vi "picture_c_labview2014.vi"() -> ()   [LabVIEW 2014]
uses:
  Program Files (x86)/National Instruments/LabVIEW 2017/instr.lib/Lake Shore 336/Lake Shore 336.lvlib
  Program Files (x86)/National Instruments/LabVIEW 2017/instr.lib/Lake Shore 336/Public/Data/Sensor Data (Single Reading).vi
  Program Files (x86)/National Instruments/LabVIEW 2017/instr.lib/Lake Shore 372/Lake Shore 372.lvlib
  <vilib>/Utility/file.llb/Write Delimited Spreadsheet (string).vi
panel:
  out "current time":timestamp format="%<%I:%M:%S %p>T"
  in  "Tab Control":T1(tab)
  out "Reading 372":bool
  out "Reading 336":bool
  out "Arduino OK":bool
  out "Nitrogen tank":waveform(dbl)(graph)={"t0"=timestamp(3512160360.4800687 s since 1904-01-01), "dt"=0.0, "Y"=[0.0]}
  out "Helium tank":waveform(dbl)[](graph)=[{"t0"=timestamp(3512160360.4800687 s since 1904-01-01), "dt"=0.0, "Y"=[0.0]}, {"t0"=timestamp(3512160360.4800687 s since 1904-01-01), "dt"=0.0, "Y"=[0.0]}]
  out "Device (red) and FAA (green)":waveform(dbl)[](graph)=[{"t0"=timestamp(3512160360.6630793 s since 1904-01-01), "dt"=0.0, "Y"=[0.0]}, {"t0"=timestamp(3512160360.6630793 s since 1904-01-01), "dt"=0.0, "Y"=[0.0]}]
  in  "Stop":bool=TRUE
  out "stopping":bool=TRUE
  out "FAA RO600":dbl caption="FAA (K)" min=0.0 max=63200000.0 step=1e-05 format="%_4f"
  out "Sample RuOx":dbl caption="Device (K)" min=0.0 max=63200000.0 step=1e-05 format="%_3f"
  out "Magnet Current (A)":dbl format="%.3f"
  out "4K Diode":dbl format="%_4f"
  out "77K Diode":dbl format="%_4f"
  out "Magnetic Field (kG)":dbl min=-601000.0 max=601000.0 step=0.0001 format="%_3f"
  in  "Auto-Ramp":bool
  in  "ramp start time":timestamp
  out "Ramp Status":string="Shutting down"
  out "Ramp State":u16(ring)=6 items=["Ramp Up", "Soak (hold)", "Ramp Down", "Ramp up to Setpoint", "Closed Loop Feedback", "Ramp down from Setpoint", "Magnet off"]
  out "Magnet Current":waveform(dbl)(graph)={"t0"=timestamp(3512160360.4800687 s since 1904-01-01), "dt"=0.0, "Y"=[0.0]}
  in  "Calculate Autoramp Time":bool
  in  "End of Ramp Temp Control":bool=TRUE
  in  "soak time (minutes)":dbl=30.0
  out "cycle time (min)":dbl format="%#_3g"
  out "Ramp down step size (mA)":dbl=1.0
  in  "setpoint (K)":dbl=0.1
  in  "Manual temp control":bool
  in  "Check Arduino":bool
  in  "ls336":refnum<visa-resource-name>="LS336"
  in  "ls372":refnum<visa-resource-name>="LS372"
  in  "Arduino":refnum<visa-resource-name>="COM4"
  out "Ramp up step size (%)":dbl=0.02
  out "max magnet value(%)":dbl=10.0
  in  "Read LS336":bool=TRUE
  in  "Read LS372":bool=TRUE
  in  "Record Temps":bool=TRUE
  in  "Timeout (ms)":i32=1000
  out "Ramp up step size (mA)":dbl=1.0
  in  "Max current (A)":dbl=9.4
  in  "thermo data path":path=path "C:/Data/temperature_log/pictureC"
  in  "Field constant (kG/A)":dbl=4.589 min=0.001 max=10.0 step=1e-05 format="%.3f"
  out "Ramp down step size (%)":dbl=0.02
  out "ramp up time (min)":dbl=60.0
  out "ramp down time (min)":dbl=60.0
  out "ramp down start time":timestamp
  in  "Ramp up rate (mA/s)":dbl=5.0
  in  "Ramp down rate (mA/s)":dbl=5.0
  in  "Heat Switch":bool
  in  "Ramp Magnet Up":bool
  in  "Ramp Magnet Down":bool
  in  "control channel":string="A"
  out "Arduino Response":string
  in  "Arduino IP":string="10.200.130.3"
  out "Arduino error":errorcluster
  out "counter":dbl
  in  "delay after ramp down (min)":dbl=20.0
  out "counter 2":dbl
  out "ramp finish time":timestamp
  out "Magnet Current (%)":dbl format="%.3f"
  out "Heater Range Set":u16(ring) items=["Off", "31.6 uA", "100 uA", "316 uA", "1.00 mA", "3.16 mA", "10.0 mA", "31.6 mA", "100 mA"]
  out "Heater Range Actual":u16(ring) items=["Off", "31.6 uA", "100 uA", "316 uA", "1.00 mA", "3.16 mA", "10.0 mA", "31.6 mA", "100 mA"]
  out "Magnet Current Multiplier":dbl=1.0
  out "Heater Range OK":bool
  out "actual Setpoint":dbl min=0.0 max=100000000.0 step=1e-06 format="%.5f"
  in  "Channel (1)":u16(ring)=1 items=["1"=1, "2"=2, "3"=3, "4"=4, "5"=5, "6"=6, "7"=7, "8"=8, "9"=9, "10"=10, "11"=11, "12"=12, "13"=13, "14"=14, "15"=15, "16"=16, "A (Control Input)"=17]
  in  "Excitation Range (5: 200 uV / 100 pA)":u16(ring)=5 items=["2.00 uV / 1.00 pA"=1, "6.32 uV / 3.16 pA"=2, "20.0 uV / 10.0 pA"=3, "63.2 uV / 31.6 pA"=4, "200 uV / 100 pA"=5, "632 uV / 316 pA"=6, "2.00 mV / 1.00 nA"=7, "6.32 mV / 3.16 nA"=8, "20.0 mV / 10.0 nA"=9, "63.2 mV / 31.6 nA"=10, "200 mV / 100 nA"=11, "632 mV / 316 nA"=12, "1.00 uA"=13, "3.16 uA"=14, "10.0 uA"=15, "31.6 uA"=16, "100 uA"=17, "316 uA"=18, "1.00 mA"=19, "3.16 mA"=20, "10.0 mA"=21, "31.6 mA"=22]
  in  "Autorange (0: Autorange off)":u16(ring) items=["Autorange off", "Autorange Current", "ROX 102B Autorange"]
  in  "Excitation  (T: On)":bool=TRUE
  in  "Excitation Mode (0: Voltage)":u16(ring) items=["Voltage", "Current"]
  in  "Resistance Range (17: 200 kOhm)":u16(ring)=17 items=["2.00 mOhm"=1, "6.32 mOhm"=2, "20.0 mOhm"=3, "63.2 mOhm"=4, "200 mOhm"=5, "632 mOhm"=6, "2.00 Ohm"=7, "6.32 Ohm"=8, "20.0 Ohm"=9, "63.2 Ohm"=10, "200 Ohm"=11, "632 Ohm"=12, "2.00 kOhm"=13, "6.32 kOhm"=14, "20.0 kOhm"=15, "63.2 kOhm"=16, "200 kOhm"=17, "632 kOhm"=18, "2.00 MOhm"=19, "6.32 MOhm"=20, "20.0 MOhm"=21, "63.2 MOhm"=22]
  in  "Heater ON/OFF":bool
  in  "Warmup Heater Power (W)":dbl min=0.0 max=10.0
  out "Magnet RTD R":dbl caption="Magnet R (Ohms)" format="%.2f"
  out "GGG RO600 R":dbl caption="GGG R (Ohms)" format="%_4f"
  out "GGG RO600":dbl caption="GGG (K)" format="%_4f"
  out "Magnet RTD":dbl caption="Magnet (K)" format="%.2f"
  out "FAA RO600 R":dbl caption="FAA R (Ohms)" min=0.0 max=63200000.0 step=1e-05 format="%_4f"
  out "Sample RuOx R":dbl caption="Device R (Ohms)" min=0.0 max=63200000.0 step=1e-05 format="%_3f"
  out "GGG":waveform(dbl)(graph)={"t0"=timestamp(3512160360.4800687 s since 1904-01-01), "dt"=0.0, "Y"=[0.0]}
  out "magnet":waveform(dbl)(graph)={"t0"=timestamp(3512160360.4800687 s since 1904-01-01), "dt"=0.0, "Y"=[0.0]}
  in  "initialize":bool
  # "PICTURE-C!"
  # "ADR CONTROL"
  # "How often to measure temps?\nDon't change this during ramps."
  # "Ramp Parameters"
  # "\"A\" for Darkness \n\"1\" for MEC"
  # "Manual ADR CONTROL"
  # "OPEN"
  # "CLOSED"
  # "Lakeshore 372"
  # "Thermometers\nUse ~ 20 uV or ~20 nA excitation for FAA and device thermometers. \nHPD recommendations (these are conservative. Scientific instruments used excitations that were 10 to 100 times higher)\nT(K)                            excitation (nA)\n.175 to 4.2                  10\n.1 to .175                    3\n<.1                              0.1\n\nDiodes get 10 uA excitation. \n\n\nIP Addresses: Palomar July 2016 \nArduino at Palomar July 2016      10.200.130.3\nLS372 at Palomar July 2016          10.200.130.1\nLS336 at Palomar July 2016           10.200.130.2\nGateway at Palomar Nov 2016     10.200.1.129\nDARKNESS lab computer (this machine)      10.200.72.36\nsubnet mask                                   255.255.0.0\n\nWhen changing IP addresses for the Lakeshores, open NIMAX and find the lakeshores under Devices and Interfaces>\nNetwork Devices. Select a Lakeshore and go to the TCP/IP tab in the right panel (tabs are at the bottom of the window.).\nChange the IP and click Validate. If the validation works, click Save.  \n\n\nKepco Front Panel\nVoltage Control = OFF\nCurrent Control = OFF\nMode = Voltage\n\nSample Heater Output from LS372 connects to Voltage Programming Input on Kepco. Red terminal on front of Kepco should\nget a voltage <0, Red magnet wire goes to OUT on back of Kepco, Blue wire goes to COM on back of Kepco.\n\n\nArduino\nTo change the ip address of the arduino, open \nC:\\Users\\kids\\Documents\\Arduino\\heatSwitch\\darkness\\heatSwitch_blackLab\\heatSwitch_blackLab.ino\nor\nC:\\Users\\kids\\Documents\\Arduino\\heatSwitch\\darkness\\heatSwitch_blackLab\\heatSwitch_palomar.ino\nand connect the arduino to this computer (darkness.physics.ucsb.edu) and upload the new file.\n\nFor debugging the UDP connection, use \nC:\\Users\\kids\\Documents\\DARKNESS_labview\\arduino_udp_test.vi"
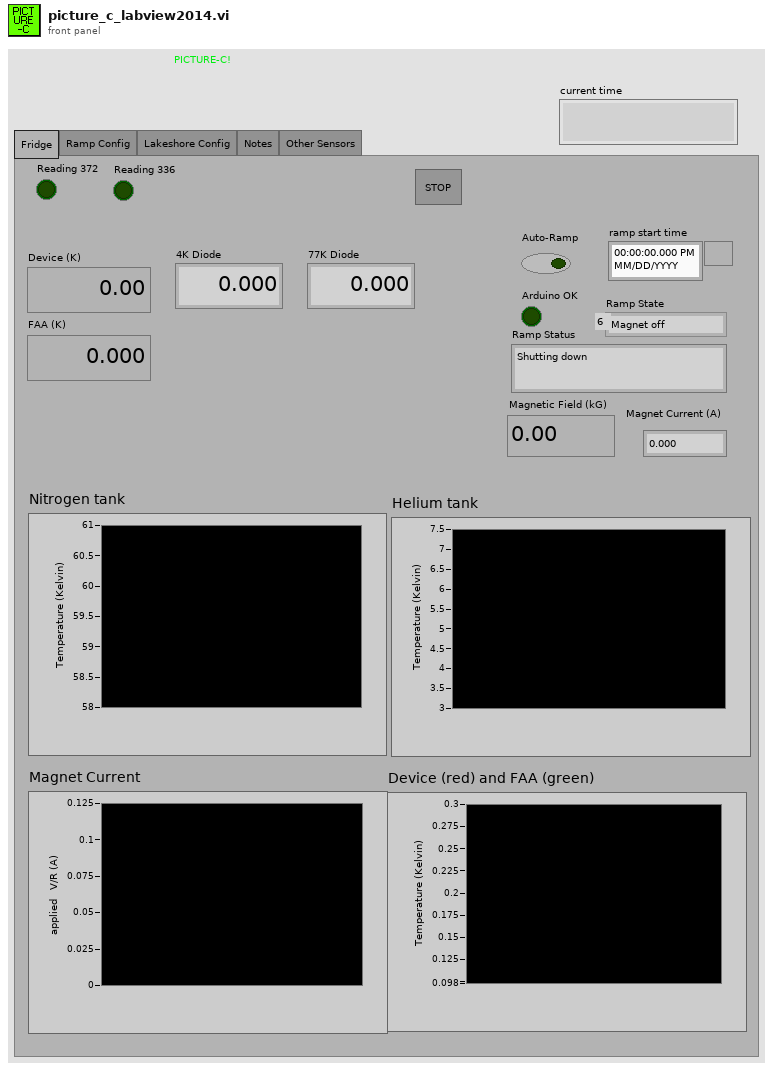
[diagram p1: front panel]
types:
  T1 = enum32{"Fridge", "Ramp Config", "Lakeshore Config", "Notes", "Other Sensors"}
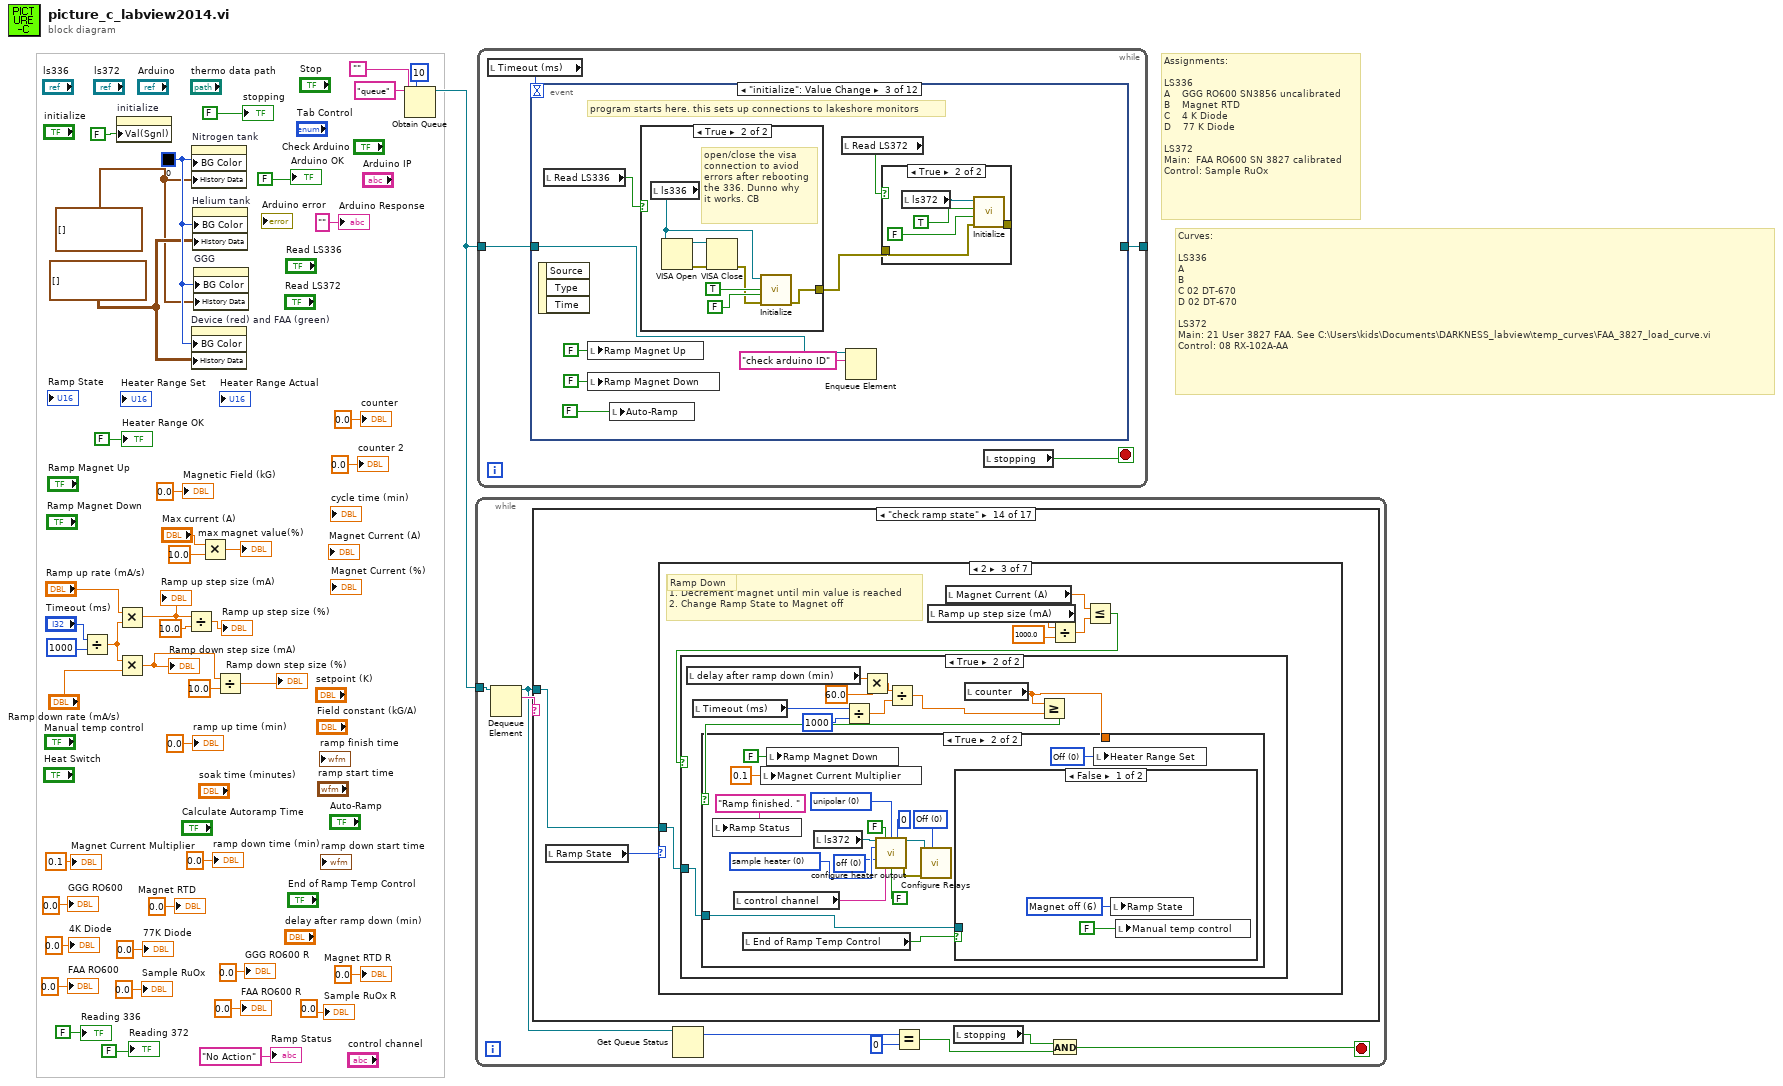
[diagram p0: block diagram]
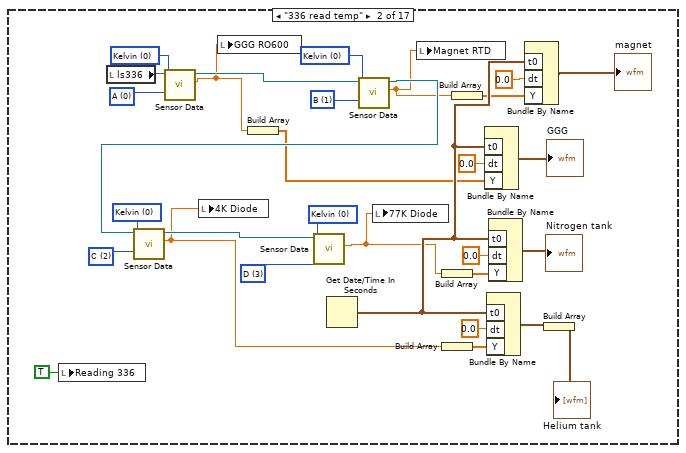
[diagram p3: hidden frame]
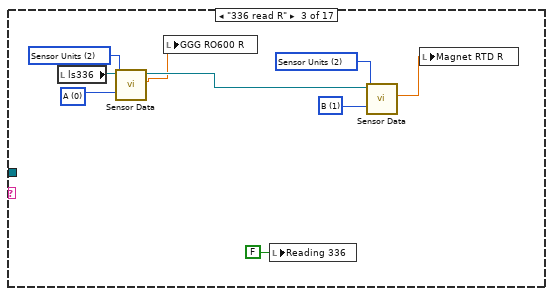
[diagram p4: hidden frame]
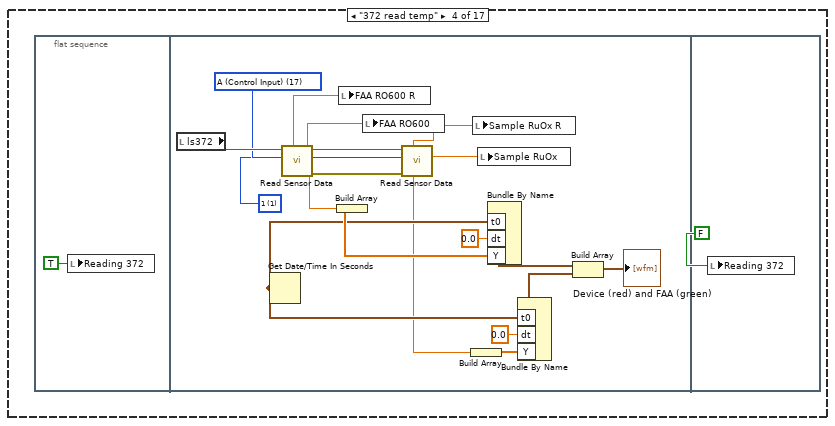
[diagram p5: hidden frame]
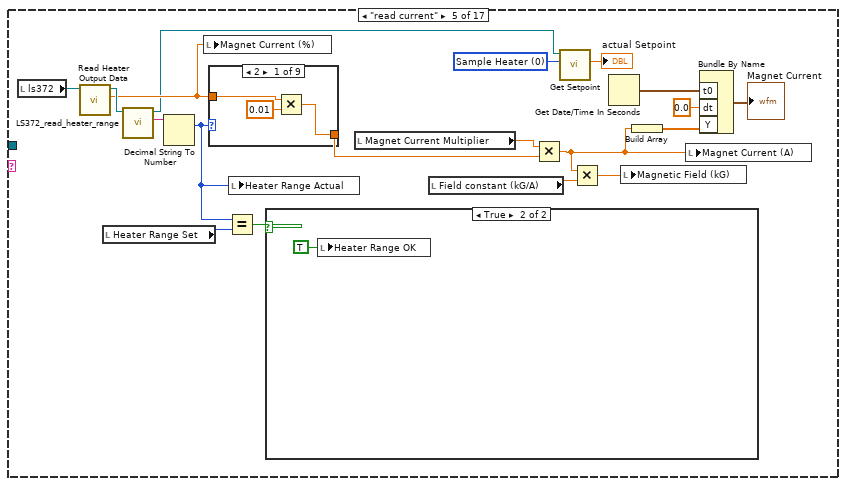
[diagram p6: hidden frame]
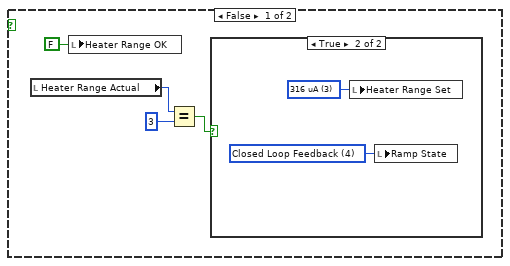
[diagram p7: hidden frame]
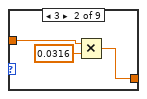
[diagram p9: hidden frame]
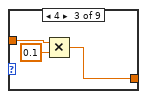
[diagram p10: hidden frame]
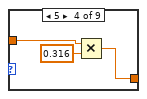
[diagram p11: hidden frame]
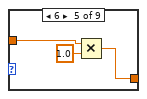
[diagram p12: hidden frame]
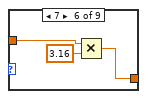
[diagram p13: hidden frame]
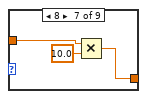
[diagram p14: hidden frame]
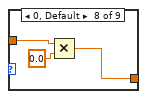
[diagram p15: hidden frame]
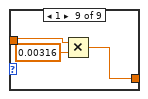
[diagram p16: hidden frame]
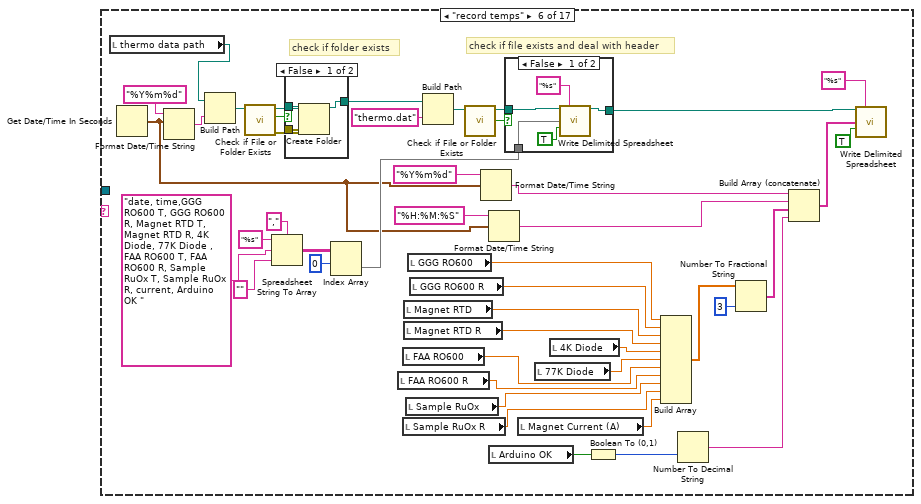
[diagram p17: hidden frame]
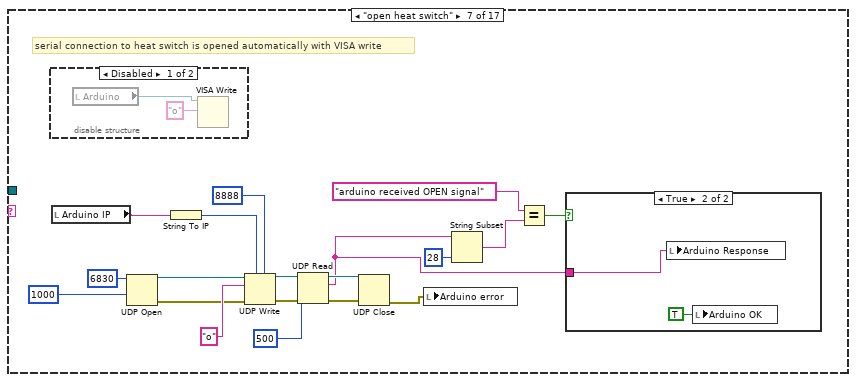
[diagram p20: hidden frame]
diagram:
  w11 = waveform(dbl)[][] [] ("History Data")
  w10 = waveform(dbl)[] [] ("History Data")
  w35 = u32 0
  # "Curves:\n\nLS336\nA\nB\nC 02 DT-670\nD 02 DT-670\n\nLS372\nMain: 21 User 3827 FAA. See C:\\Users\\kids\\Documents\\DARKNESS_labview\\temp_curves\\FAA_3827_load_curve.vi\nControl: 08 RX-102A-AA"
  # "Assignments:\n\nLS336\nA    GGG RO600 SN3856 uncalibrated\nB    Magnet RTD\nC    4 K Diode\nD    77 K Diode\n\nLS372\nMain:  FAA RO600 SN 3827 calibrated\nControl: Sample RuOx"
  n1 = Divide(x="Timeout (ms)", y=1000) -> (x/y=w15:dbl)
  n2 = property on="initialize" class="Bool (strict)"("Val(Sgnl)"=FALSE ("Boolean")) -> ()  [unwired: 2 in, 2 out]
  n3 = Multiply(x="Ramp up rate (mA/s)", y=w15) -> (x*y=w12:dbl)
  "Ramp up step size (mA)" <- w12
  n4 = Multiply(x=w15, y="Ramp down rate (mA/s)") -> (x*y=w13:dbl)
  "Ramp down step size (mA)" <- w13
  n5 = Divide(x=w12, y=10.0) -> (x/y=→"Ramp up step size (%)":dbl)
  n6 = property on="Nitrogen tank" class="WFChart (strict)"("BG Color"=w35, "History Data"=w10) -> ()  [unwired: 2 in, 2 out]
  n7 = property on="Device (red) and FAA (green)" class="WFChart (strict)"("BG Color"=w35, "History Data"=w11) -> ()  [unwired: 2 in, 2 out]
  n8 = property on="Helium tank" class="WFChart (strict)"("BG Color"=w35, "History Data"=w11) -> ()  [unwired: 2 in, 2 out]
  n9 = property on="GGG" class="WFChart (strict)"("BG Color"=w35, "History Data"=w10) -> ()  [unwired: 2 in, 2 out]
  n10 = Multiply(x="Max current (A)", y=10.0) -> (x*y=→"max magnet value(%)":dbl)
  n11 = Divide(x=w13, y=10.0) -> (x/y=→"Ramp down step size (%)":dbl)
  n12 = Obtain Queue(max queue size (-1, unlimited)=10, name (unnamed)="queue", element data type="") -> (queue out=w43:refnum<queue>)  [unwired: 2 in, 2 out]
  n13 = while {
    tunnel: w43 -> [w53]
    stop <- w47 stop-if-true
    n14 = Dequeue Element(queue=w53) -> (queue out=w46:refnum<queue>, element=w52:string)  [unwired: 2 in, 2 out]
    n15 = case shown="\"check ramp state\"" w52 {
      tunnel: w46 -> [_ _ _ _ _ _ _ _ _ _ _ _ _ w477 _ _ _]
      frame "False", Default {
      }
      frame "336 read temp" {
        w74 = u16 0 items=["Kelvin", "Celsius", "Sensor Units"] ("Data Source (0:Kelvin)")
        w75 = u16 3 items=["A", "B", "C", "D"] ("Input (0:A)")
        w77 = u16 0 items=["Kelvin", "Celsius", "Sensor Units"] ("Data Source (0:Kelvin)")
        w78 = u16 2 items=["A", "B", "C", "D"] ("Input (0:A)")
        w80 = u16 0 items=["Kelvin", "Celsius", "Sensor Units"] ("Data Source (0:Kelvin)")
        w81 = u16 1 items=["A", "B", "C", "D"] ("Input (0:A)")
        w82 = u16 0 items=["Kelvin", "Celsius", "Sensor Units"] ("Data Source (0:Kelvin)")
        w83 = u16 0 items=["A", "B", "C", "D"] ("Input (0:A)")
        n16 = local write "Reading 336"(TRUE ("Reading 336")) -> ()
        n17 = local read "ls336"() -> (w84:refnum<visa-resource-name>)
        n18 = call-poly "Sensor Data.vi"("Data Source (0:Kelvin)"=w82, "Input (0:A)"=w83, "VISA resource name"=w84) -> ("Sensor Data"=w62:dbl, "VISA resource name out"=w79:refnum<visa-resource-name>)  [unwired: 6 in, 1 out]
        n19 = local write "GGG RO600"(w62) -> ()
        n20 = Build Array(w62) -> (w63:dbl[])
        n21 = Get Date/Time In Seconds() -> (seconds since 1Jan1904=w67:timestamp)
        n22 = call-poly "Sensor Data.vi"("Data Source (0:Kelvin)"=w80, "Input (0:A)"=w81, "VISA resource name"=w79) -> ("Sensor Data"=w61:dbl, "VISA resource name out"=w76:refnum<visa-resource-name>)  [unwired: 6 in, 1 out]
        n23 = call-poly "Sensor Data.vi"("Data Source (0:Kelvin)"=w77, "Input (0:A)"=w78, "VISA resource name"=w76) -> ("Sensor Data"=w60:dbl, "VISA resource name out"=w73:refnum<visa-resource-name>)  [unwired: 6 in, 1 out]
        n24 = local write "4K Diode"(w60) -> ()
        n25 = call-poly "Sensor Data.vi"("Data Source (0:Kelvin)"=w74, "Input (0:A)"=w75, "VISA resource name"=w73) -> ("Sensor Data"=w59:dbl)  [unwired: 6 in, 2 out]
        n26 = local write "77K Diode"(w59) -> ()
        n27 = local write "Magnet RTD"(w61) -> ()
        n28 = Build Array(w59) -> (w70:dbl[])
        n29 = Build Array(w60) -> (w69:dbl[])
        n30 = Build Array(w61) -> (w64:dbl[])
        n31 = Bundle By Name("t0"=w67, "dt"=0.0, "Y"=w63) -> (→"GGG":waveform(dbl))  [unwired: 1 in]
        n32 = Bundle By Name("t0"=w67, "dt"=0.0, "Y"=w69) -> (w57:waveform(dbl))  [unwired: 1 in]
        n33 = Bundle By Name("t0"=w67, "dt"=0.0, "Y"=w70) -> (→"Nitrogen tank":waveform(dbl))  [unwired: 1 in]
        n34 = Bundle By Name("t0"=w67, "dt"=0.0, "Y"=w64) -> (→"magnet":waveform(dbl))  [unwired: 1 in]
        n35 = Build Array(w57) -> (→"Helium tank":waveform(dbl)[])
      }
      frame "336 read R" {
        w89 = u16 2 items=["Kelvin", "Celsius", "Sensor Units"] ("Data Source (0:Kelvin)")
        w90 = u16 1 items=["A", "B", "C", "D"] ("Input (0:A)")
        w91 = u16 2 items=["Kelvin", "Celsius", "Sensor Units"] ("Data Source (0:Kelvin)")
        w92 = u16 0 items=["A", "B", "C", "D"] ("Input (0:A)")
        n36 = local read "ls336"() -> (w93:refnum<visa-resource-name>)
        n37 = call-poly "Sensor Data.vi"("Data Source (0:Kelvin)"=w91, "Input (0:A)"=w92, "VISA resource name"=w93) -> ("Sensor Data"=w87:dbl, "VISA resource name out"=w88:refnum<visa-resource-name>)  [unwired: 6 in, 1 out]
        n38 = local write "GGG RO600 R"(w87) -> ()
        n39 = local write "Reading 336"(FALSE ("Reading 336")) -> ()
        n40 = call-poly "Sensor Data.vi"("Data Source (0:Kelvin)"=w89, "Input (0:A)"=w90, "VISA resource name"=w88) -> ("Sensor Data"=w86:dbl)  [unwired: 6 in, 2 out]
        n41 = local write "Magnet RTD R"(w86) -> ()
      }
      frame "372 read temp" {
        n42 = flat-sequence {
          frame #0 {
            n43 = local write "Reading 372"(TRUE ("Reading 372")) -> ()
          }
          frame #1 {
            w95 = u16 1 items=["1"=1, "2"=2, "3"=3, "4"=4, "5"=5, "6"=6, "7"=7, "8"=8, "9"=9, "10"=10, "11"=11, "12"=12, "13"=13, "14"=14, "15"=15, "16"=16, "A (Control Input)"=17] ("Channel (1:1)")
            w96 = u16 17 items=["1"=1, "2"=2, "3"=3, "4"=4, "5"=5, "6"=6, "7"=7, "8"=8, "9"=9, "10"=10, "11"=11, "12"=12, "13"=13, "14"=14, "15"=15, "16"=16, "A (Control Input)"=17] ("Channel (1:1)")
            n44 = local read "ls372"() -> (w111:refnum<visa-resource-name>)
            n45 = Get Date/Time In Seconds() -> (seconds since 1Jan1904=w101:timestamp)
            n46 = call "Read Sensor Data.vi"("Channel (1:1)"=w95, "VISA resource name"=w111) -> ("error out"=w109:errorcluster, "Kelvin Reading"=w100:dbl, "Resistance Reading"=w97:dbl, "VISA resource name out"=w110:refnum<visa-resource-name>)  [unwired: 4 in, 2 out]
            n47 = Build Array(w100) -> (w106:dbl[])
            n48 = local write "FAA RO600 R"(w97) -> ()
            n49 = local write "FAA RO600"(w100) -> ()
            n50 = call "Read Sensor Data.vi"("error in (no error)"=w109, "Channel (1:1)"=w96, "VISA resource name"=w110) -> ("Kelvin Reading"=w99:dbl, "Resistance Reading"=w98:dbl)  [unwired: 3 in, 4 out]
            n51 = Build Array(w99) -> (w103:dbl[])
            n52 = local write "Sample RuOx R"(w98) -> ()
            n53 = local write "Sample RuOx"(w99) -> ()
            n54 = Bundle By Name("t0"=w101, "dt"=0.0, "Y"=w106) -> (w107:waveform(dbl))  [unwired: 1 in]
            n55 = Bundle By Name("t0"=w101, "dt"=0.0, "Y"=w103) -> (w102:waveform(dbl))  [unwired: 1 in]
            n56 = Build Array(w107, w102) -> (→"Device (red) and FAA (green)":waveform(dbl)[])
          }
          frame #2 {
            n57 = local write "Reading 372"(FALSE ("Reading 372")) -> ()
          }
        }
      }
      frame "read current" {
        w119 = u16 0 items=["Sample Heater", "Warm-up Heater (Output 1)"] ("Output (0:Sample Heater)")
        n58 = local read "ls372"() -> (w129:refnum<visa-resource-name>)
        n59 = call "Read Heater Output Data.vi"("VISA resource name"=w129) -> ("Heater Output"=w123:dbl, "VISA resource name out"=w128:refnum<visa-resource-name>)  [unwired: 8 in, 1 out]
        n60 = local read "Heater Range Set"() -> (w125:u16)
        n61 = call "LS372_read_heater_range.vi"("VISA resource name"=w128) -> ("heater range"=w127:string, "VISA resource name out"=w118:refnum<visa-resource-name>)  [unwired: 9 in]
        n62 = Decimal String To Number(string=w127) -> (number=w126:i32)  [unwired: 2 in, 1 out]
        n63 = local write "Magnet Current (%)"(w123) -> ()
        n64 = case shown="2" w126 {
          tunnel: [w139 w142 w145 w148 w151 w154 w157 w160 w164] -> w121
          tunnel: w123 -> [w140 w143 w146 w149 w152 w155 w158 w161 w163]
          frame 2 {
            n65 = Multiply(x=w140, y=0.01) -> (x*y=w139:dbl)
          }
          frame 3 {
            n66 = Multiply(x=w143, y=0.0316) -> (x*y=w142:dbl)
          }
          frame 4 {
            n67 = Multiply(x=w146, y=0.1) -> (x*y=w145:dbl)
          }
          frame 5 {
            n68 = Multiply(x=w149, y=0.316) -> (x*y=w148:dbl)
          }
          frame 6 {
            n69 = Multiply(x=w152, y=1.0) -> (x*y=w151:dbl)
          }
          frame 7 {
            n70 = Multiply(x=w155, y=3.16) -> (x*y=w154:dbl)
          }
          frame 8 {
            n71 = Multiply(x=w158, y=10.0) -> (x*y=w157:dbl)
          }
          frame 0, Default {
            n72 = Multiply(x=w161, y=0.0) -> (x*y=w160:dbl)
          }
          frame 1 {
            n73 = Multiply(x=w163, y=0.00316) -> (x*y=w164:dbl)
          }
        }
        n74 = Equal?(x=w126, y=w125) -> (x = y?=w124:bool)
        n75 = local write "Heater Range Actual"(w126) -> ()
        n76 = case shown="True" w124 {
          frame False {
            n77 = local read "Heater Range Actual"() -> (w132:u16)
            n78 = local write "Heater Range OK"(FALSE ("Heater Range OK")) -> ()
            n79 = Equal?(x=w132, y=u16 3) -> (x = y?=w134:bool)
            n80 = case shown="True" w134 {
              frame False {
              }
              frame True {
                w136 = u16 3 items=["Off", "31.6 uA", "100 uA", "316 uA", "1.00 mA", "3.16 mA", "10.0 mA", "31.6 mA", "100 mA"] ("Heater Range Set")
                w137 = u16 4 items=["Ramp Up", "Soak (hold)", "Ramp Down", "Ramp up to Setpoint", "Closed Loop Feedback", "Ramp down from Setpoint", "Magnet off"] ("Ramp State")
                n81 = local write "Heater Range Set"(w136) -> ()
                n82 = local write "Ramp State"(w137) -> ()
              }
            }
          }
          frame True {
            n83 = local write "Heater Range OK"(TRUE ("Heater Range OK")) -> ()
          }
        }
        n84 = local read "Magnet Current Multiplier"() -> (w122:dbl)
        n85 = local read "Field constant (kG/A)"() -> (w131:dbl)
        n86 = Multiply(x=w122, y=w121) -> (x*y=w113:dbl)
        n87 = call "Get Setpoint.vi"("Output (0:Sample Heater)"=w119, "VISA resource name"=w118) -> ("Setpoint (0.00000E+0)"=→"actual Setpoint":dbl)  [unwired: 7 in, 2 out]
        n88 = Multiply(x=w113, y=w131) -> (x*y=w130:dbl)
        n89 = Get Date/Time In Seconds() -> (seconds since 1Jan1904=w117:timestamp)
        n90 = local write "Magnetic Field (kG)"(w130) -> ()
        n91 = Build Array(w113) -> (w116:dbl[])
        n92 = local write "Magnet Current (A)"(w113) -> ()
        n93 = Bundle By Name("t0"=w117, "dt"=0.0, "Y"=w116) -> (→"Magnet Current":waveform(dbl))  [unwired: 1 in]
      }
      frame "record temps" {
        # "check if file exists and deal with header"
        # "check if folder exists"
        n94 = local read "thermo data path"() -> (w186:path)
        n95 = Get Date/Time In Seconds() -> (seconds since 1Jan1904=w176:timestamp)
        n96 = Format Date/Time String(time format string (%c)="%Y%m%d", seconds (now)=w176) -> (date/time string=w198:string)  [unwired: 1 in]
        n97 = Build Path(base path=w186, name or relative path=w198) -> (appended path=w201:path)
        n98 = call <vilib>:"Check if File or Folder Exists.vi"("path"=w201) -> ("error out"=w204:errorcluster, "file or folder exists?"=w203:bool, "dup path"=w202:path)  [unwired: 8 in]
        n99 = Spreadsheet String To Array(delimiter (Tab)=",", format string="%s", spreadsheet string="date, time,GGG RO600 T, GGG RO600 R, Magnet RTD T, Magnet RTD R, 4K Diode, 77K Diode , FAA RO600 T, FAA RO600 R, Sample RuOx T, Sample RuOx R, current, Arduino OK ", array type (2D Dbl)="") -> (array=w184:string[][])
        n100 = case shown="False" w203 {
          tunnel: w202 -> [w219 w220]
          tunnel: w204 -> [w218 _]
          tunnel: [w217 w220] -> w205
          frame False {
            n101 = Create Folder(path (use dialog)=w219, error in=w218) -> (created path=w217:path)  [unwired: 1 in, 2 out]
          }
          frame True {
          }
        }
        n102 = Index Array(array=w184, index (row)=0) -> (element=w178:string[])  [unwired: 1 in]
        n103 = local read "FAA RO600 R"() -> (w189:dbl)
        n104 = local read "FAA RO600"() -> (w190:dbl)
        n105 = local read "Sample RuOx R"() -> (w187:dbl)
        n106 = local read "Magnet RTD"() -> (w194:dbl)
        n107 = local read "Magnet RTD R"() -> (w193:dbl)
        n108 = local read "Sample RuOx"() -> (w188:dbl)
        n109 = local read "GGG RO600"() -> (w210:dbl)
        n110 = local read "GGG RO600 R"() -> (w195:dbl)
        n111 = Build Path(base path=w205, name or relative path="thermo.dat") -> (appended path=w206:path)
        n112 = call <vilib>:"Check if File or Folder Exists.vi"("path"=w206) -> ("file or folder exists?"=w207:bool, "dup path"=w208:path)  [unwired: 8 in, 1 out]
        n113 = Format Date/Time String(time format string (%c)="%Y%m%d", seconds (now)=w176) -> (date/time string=w174:string)  [unwired: 1 in]
        n114 = Format Date/Time String(time format string (%c)="%H:%M:%S", seconds (now)=w176) -> (date/time string=w173:string)  [unwired: 1 in]
        n115 = local read "Arduino OK"() -> (w185:bool)
        n116 = case shown="False" w207 {
          tunnel: [w212 w216] -> w209
          tunnel: w208 -> [w213 w216]
          tunnel: w178 -> [w211 _]
          frame False {
            n117 = call-poly <vilib>:"Write Delimited Spreadsheet.vi"("file path (dialog if empty)"=w213, "format (%s)"="%s" ("format (%.3f)"), "1D data"=w211, "append to file? (new file:F)"=TRUE) -> ("new file path (Not A Path if cancelled)"=w212:path)  [unwired: 10 in, 1 out]
          }
          frame True {
          }
        }
        n118 = local read "Magnet Current (A)"() -> (w196:dbl)
        n119 = local read "77K Diode"() -> (w191:dbl)
        n120 = local read "4K Diode"() -> (w192:dbl)
        n121 = Boolean To (0,1)(Boolean=w185) -> (0, 1=w167:i16)
        n122 = Build Array(w210, w195, w194, w193, w192, w191, w190, w189, w188, w187, w196) -> (w171:dbl[])
        n123 = Number To Decimal String(number=w167) -> (decimal integer string=w166:string)  [unwired: 1 in]
        n124 = Number To Fractional String(number=w171, precision (6)=i16 3) -> (F-format string=w170:string[])  [unwired: 2 in]
        n125 = Build Array (concatenate)(w174, w173, w170, w166) -> (w169:string[])
        n126 = call-poly <vilib>:"Write Delimited Spreadsheet.vi"("file path (dialog if empty)"=w209, "format (%s)"="%s" ("format (%.3f)"), "1D data"=w169, "append to file? (new file:F)"=TRUE) -> ()  [unwired: 10 in, 2 out]
      }
      frame "open heat switch" {
        # "serial connection to heat switch is opened automatically with VISA write"
        n127 = disable-structure shown="Disabled" {
          frame Disabled {
            n128 = local read "Arduino"() -> (w244:refnum<visa-resource-name>)
            n129 = VISA Write(VISA resource name=w244, write buffer="o") -> ()  [unwired: 1 in, 3 out]
          }
          frame Enabled {
          }
        }
        n130 = local read "Arduino IP"() -> (w228:string)
        n131 = UDP Open(9:1000 ("timeout ms (25000)"), 11:u16 6830 ("port")) -> (port=w230:refnum<k16>, 0:w231:errorcluster)  [unwired: 3 in, 1 out]
        n132 = String To IP(1:w228) -> (0:w232:u32)
        n133 = UDP Write(address=w232, port or service name=u16 8888, connection ID=w230, data in="o", 8:w231) -> (error out=w236:errorcluster, 3:w235:refnum<k16>)  [unwired: 1 in]
        n134 = UDP Read(connection ID=w235, timeout ms (25000)=500, 8:w236) -> (data out=w221:string, error out=w239:errorcluster, 3:w238:refnum<k16>)  [unwired: 1 in, 2 out]
        n135 = UDP Close(connection ID=w238, 8:w239) -> (error out=w227:errorcluster)  [unwired: 1 out]
        n136 = local write "Arduino error"(w227) -> ()
        n137 = String Subset(string=w221, length (rest)=28 ("length (rest)")) -> (substring=w222:string)  [unwired: 1 in]
        n138 = Equal?(x="arduino received OPEN signal", y=w222) -> (x = y?=w225:bool)
        n139 = case shown="True" w225 {
          tunnel: w221 -> [_ w242]
          frame False {
            n140 = local write "Arduino Response"("did not respond" ("Arduino Response")) -> ()
            n141 = local write "Arduino OK"(FALSE ("Arduino OK")) -> ()
          }
          frame True {
            n142 = local write "Arduino Response"(w242) -> ()
            n143 = local write "Arduino OK"(TRUE ("Arduino OK")) -> ()
          }
        }
      }
      frame "close heat switch" {
        n144 = local read "Ramp State"() -> (w246:u16)
        n145 = local read "Arduino IP"() -> (w254:string)
        n146 = UDP Open(9:1000 ("timeout ms (25000)"), 11:u16 6830 ("port")) -> (port=w256:refnum<k16>, 0:w257:errorcluster)  [unwired: 3 in, 1 out]
        n147 = case shown="4" w246 {
          frame 0, Default {
          }
          frame 4 {
            w276 = u16 0 items=["unipolar", "bipolar"] ("polarity")
            w277 = u16 0 items=["Off", "31.6 uA", "100 uA", "316 uA", "1.00 mA", "3.16 mA", "10.0 mA", "31.6 mA", "100 mA"] ("Heater Range Set")
            w278 = u16 6 items=["Ramp Up", "Soak (hold)", "Ramp Down", "Ramp up to Setpoint", "Closed Loop Feedback", "Ramp down from Setpoint", "Magnet off"] ("Ramp State")
            w280 = u16 0 items=["sample heater", "output 1 (warm-up heater) ", "output 2 (analog/still)"] ("Output (0: sample heater)")
            w279 = u16 0 items=["off", "monitor out", "open loop (manual)", "zone", "still", "closed loop (PID)", "warmup"] ("mode")
            n148 = local read "ls372"() -> (w270:refnum<visa-resource-name>)
            n149 = Get Date/Time String() -> (time string=w268:string)  [unwired: 3 in, 1 out]
            n150 = Concatenate Strings("heat switch closed at " ("Ramp Status"), w268) -> (w267:string)
            n151 = call "Configure Setpoint.vi"("Setpoint (0.00000E+0)"=0.01, "VISA resource name"=w270) -> ("VISA resource name out"=w269:refnum<visa-resource-name>)  [unwired: 8 in, 1 out]
            n152 = local read "control channel"() -> (w272:string)
            n153 = local write "Ramp Status"(w267) -> ()
            n154 = call "configure heater output.vi"("VISA resource name"=w269, "power up enable"=FALSE, "polarity"=w276, "delay"=0, "Output (0: sample heater)"=w280, "mode"=w279, "input/channel"=w272, "filter"=FALSE) -> ()  [unwired: 6 in, 2 out]
            n155 = local write "Heater Range Set"(w277) -> ()
            n156 = local write "Ramp State"(w278) -> ()
          }
        }
        n157 = String To IP(1:w254) -> (0:w258:u32)
        n158 = UDP Write(address=w258, port or service name=u16 8888, connection ID=w256, data in="c", 8:w257) -> (error out=w262:errorcluster, 3:w261:refnum<k16>)  [unwired: 1 in]
        n159 = UDP Read(connection ID=w261, timeout ms (25000)=500, 8:w262) -> (data out=w247:string, error out=w265:errorcluster, 3:w264:refnum<k16>)  [unwired: 1 in, 2 out]
        n160 = UDP Close(connection ID=w264, 8:w265) -> (error out=w253:errorcluster)  [unwired: 1 out]
        n161 = String Subset(string=w247, length (rest)=29 ("length (rest)")) -> (substring=w248:string)  [unwired: 1 in]
        n162 = local write "Arduino error"(w253) -> ()
        n163 = Equal?(x="arduino received CLOSE signal", y=w248) -> (x = y?=w251:bool)
        n164 = case shown="True" w251 {
          tunnel: w247 -> [_ w283]
          frame False {
            n165 = local write "Arduino Response"("did not respond" ("Arduino Response")) -> ()
            n166 = local write "Arduino OK"(FALSE ("Arduino OK")) -> ()
          }
          frame True {
            n167 = local write "Arduino Response"(w283) -> ()
            n168 = local write "Arduino OK"(TRUE ("Arduino OK")) -> ()
          }
        }
      }
      frame "check arduino ID" {
        # "string received from arduino probably has \\r\\n or \nor something at end, so only look at first 25 \ncharacters"
        n169 = local read "Arduino IP"() -> (w293:string)
        n170 = String To IP(1:w293) -> (0:w297:u32)
        n171 = UDP Open(9:1000 ("timeout ms (25000)"), 11:u16 8888 ("port")) -> (port=w295:refnum<k16>, 0:w296:errorcluster)  [unwired: 3 in, 1 out]
        n172 = UDP Write(address=w297, port or service name=u16 8888, connection ID=w295, data in="I", 8:w296) -> (error out=w300:errorcluster, 3:w299:refnum<k16>)  [unwired: 1 in]
        n173 = UDP Read(connection ID=w299, timeout ms (25000)=500, 8:w300) -> (data out=w289:string, error out=w303:errorcluster, 3:w302:refnum<k16>)  [unwired: 1 in, 2 out]
        n174 = UDP Close(connection ID=w302, 8:w303) -> (error out=w286:errorcluster)  [unwired: 1 out]
        n175 = String Subset(string=w289, length (rest)=25 ("length (rest)")) -> (substring=w287:string)  [unwired: 1 in]
        n176 = local write "Arduino error"(w286) -> ()
        n177 = Equal?(x="arduino says hello world!", y=w287) -> (x = y?=w290:bool)
        n178 = case shown="False" w290 {
          tunnel: w289 -> [_ w307]
          frame False {
            n179 = local write "Arduino Response"("did not respond" ("Arduino Response")) -> ()
            n180 = local write "Arduino OK"(FALSE ("Arduino OK")) -> ()
          }
          frame True {
            n181 = local write "Arduino Response"(w307) -> ()
            n182 = local write "Arduino OK"(TRUE ("Arduino OK")) -> ()
          }
        }
      }
      frame "initialize ramp up" {
        w311 = u16 1 items=["Off", "On", "Alarms", "Sample Heater Zone", "Warmup Heater Zone"] ("Relay Mode (0: Off)")
        w323 = u16 0 items=["sample heater", "output 1 (warm-up heater) ", "output 2 (analog/still)"] ("Output (0: sample heater)")
        w319 = u16 0 items=["unipolar", "bipolar"] ("polarity")
        w317 = u16 2 items=["off", "monitor out", "open loop (manual)", "zone", "still", "closed loop (PID)", "warmup"] ("mode")
        w316 = u16 0 items=["sample heater", "output 1 (warm-up heater) ", "output 2 (analog/still)"] ("Output (0: sample heater)")
        # "Start the magnet ramping up. Check whether starting ramp from 0 (what if labview crashes while\nmagnet is ramping up?)"
        n183 = local read "Ramp up step size (mA)"() -> (w329:dbl)
        n184 = local read "ls372"() -> (w328:refnum<visa-resource-name>)
        n185 = call "Read Heater Output Data.vi"("VISA resource name"=w328) -> ("error out"=w315:errorcluster, "Heater Output"=w332:dbl, "VISA resource name out"=w314:refnum<visa-resource-name>)  [unwired: 8 in]
        n186 = Divide(x=w329, y=100.0) -> (x/y=w327:dbl)
        n187 = local write "Magnet Current Multiplier"(25.66 ("Magnet Current Multiplier")) -> ()
        n188 = Less Or Equal?(x=w332, y=w327) -> (x <= y?=w330:bool)
        n189 = Select(t=0.0, s=w330, f=w332) -> (s? t:f=w313:dbl)
        n190 = local read "Heater Range Set"() -> (w312:u16)
        n191 = call "configure heater output.vi"("VISA resource name"=w314, "power up enable"=FALSE, "polarity"=w319, "delay"=0, "Output (0: sample heater)"=w316, "mode"=w317, "error in (no error)"=w315, "input/channel"="A", "filter"=FALSE) -> ("VISA resource name out"=w324:refnum<visa-resource-name>, "error out"=w325:errorcluster)  [unwired: 5 in]
        n192 = call "Configure Control Parameters.vi"("VISA resource name"=w324, "Output (0: sample heater)"=w323, "Manual Output (0.000%)"=w313, "Heater Range (0: Off)"=w312, "error in (no error)"=w325) -> ("VISA resource name out"=w310:refnum<visa-resource-name>, "error out"=w309:errorcluster)  [unwired: 9 in]
        n193 = call "Configure Relays.vi"("Relay Mode (0: Off)"=w311, "error in (no error)"=w309, "VISA resource name"=w310) -> ()  [unwired: 7 in, 2 out]
      }
      frame "set up autoramp times" {
        n194 = local read "current time"() -> (w334:timestamp)
        n195 = local read "ramp start time"() -> (w333:timestamp)
        n196 = Greater?(x=w334, y=w333) -> (0:w335:bool)
        n197 = case shown="True" w335 {
          frame True {
            n198 = Get Date/Time In Seconds() -> (seconds since 1Jan1904=w369:timestamp)
            n199 = local read "Ramp down rate (mA/s)"() -> (w348:dbl)
            n200 = local read "Max current (A)"() -> (w355:dbl)
            n201 = local read "Ramp up rate (mA/s)"() -> (w352:dbl)
            n202 = local read "Timeout (ms)"() -> (w367:i32)
            n203 = local read "Timeout (ms)"() -> (w362:i32)
            n204 = local read "Max current (A)"() -> (w349:dbl)
            n205 = Add(x=w369, y=10.0) -> (x+y=w342:timestamp)
            n206 = local write "ramp start time"(w342) -> ()
            n207 = Divide(x=w367, y=1000) -> (x/y=w365:dbl)
            n208 = Divide(x=w362, y=1000) -> (x/y=w364:dbl)
            n209 = Multiply(x=w355, y=1000.0) -> (x*y=w353:dbl)
            n210 = Multiply(x=w349, y=1000.0) -> (x*y=w351:dbl)
            n211 = Divide(x=w353, y=w352) -> (x/y=w340:dbl)
            n212 = Multiply(x=w352, y=w365) -> (x*y=w357:dbl)
            n213 = Multiply(x=w348, y=w364) -> (x*y=w356:dbl)
            n214 = Divide(x=w351, y=w348) -> (x/y=w337:dbl)
            n215 = Divide(x=w356, y=10.0) -> (x/y=w359:dbl)
            n216 = Divide(x=w357, y=10.0) -> (x/y=w358:dbl)
            n217 = local write "Ramp up step size (mA)"(w357) -> ()
            n218 = local write "Ramp down step size (mA)"(w356) -> ()
            n219 = local write "Ramp down step size (%)"(w359) -> ()
            n220 = Divide(x=w340, y=60.0) -> (x/y=w341:dbl)
            n221 = local write "Ramp up step size (%)"(w358) -> ()
            n222 = Divide(x=w337, y=60.0) -> (x/y=w338:dbl)
            n223 = local write "ramp up time (min)"(w341) -> ()
            n224 = local write "ramp down time (min)"(w338) -> ()
            n225 = local read "soak time (minutes)"() -> (w347:dbl)
            n226 = local write "Ramp Status"("Current time is greater than Start Time! Starting ramp in 10 seconds" ("AutoRamp Status")) -> ()
            n227 = Multiply(x=w347, y=60.0) -> (x*y=w345:dbl)
            n228 = Add(x=w345, y=w340) -> (x+y=w343:dbl)
            n229 = Add(x=w343, y=w342) -> (x+y=w344:timestamp)
            n230 = local write "ramp down start time"(w344) -> ()
          }
          frame False {
            n231 = local read "Ramp down rate (mA/s)"() -> (w388:dbl)
            n232 = local read "Max current (A)"() -> (w395:dbl)
            n233 = local read "Ramp up rate (mA/s)"() -> (w392:dbl)
            n234 = local read "Timeout (ms)"() -> (w407:i32)
            n235 = local read "Timeout (ms)"() -> (w402:i32)
            n236 = local read "Max current (A)"() -> (w389:dbl)
            n237 = Divide(x=w407, y=1000) -> (x/y=w405:dbl)
            n238 = Multiply(x=w395, y=1000.0) -> (x*y=w393:dbl)
            n239 = Divide(x=w402, y=1000) -> (x/y=w404:dbl)
            n240 = Multiply(x=w389, y=1000.0) -> (x*y=w391:dbl)
            n241 = Divide(x=w393, y=w392) -> (x/y=w378:dbl)
            n242 = Multiply(x=w392, y=w405) -> (x*y=w397:dbl)
            n243 = Multiply(x=w388, y=w404) -> (x*y=w396:dbl)
            n244 = Divide(x=w391, y=w388) -> (x/y=w375:dbl)
            n245 = Divide(x=w378, y=60.0) -> (x/y=w379:dbl)
            n246 = Divide(x=w396, y=10.0) -> (x/y=w399:dbl)
            n247 = Divide(x=w397, y=10.0) -> (x/y=w398:dbl)
            n248 = local write "Ramp down step size (mA)"(w396) -> ()
            n249 = local write "Ramp up step size (mA)"(w397) -> ()
            n250 = local write "ramp up time (min)"(w379) -> ()
            n251 = local write "Ramp down step size (%)"(w399) -> ()
            n252 = local write "Ramp up step size (%)"(w398) -> ()
            n253 = Divide(x=w375, y=60.0) -> (x/y=w376:dbl)
            n254 = local write "ramp down time (min)"(w376) -> ()
            n255 = local read "soak time (minutes)"() -> (w387:dbl)
            n256 = local read "delay after ramp down (min)"() -> (w372:dbl)
            n257 = local write "Ramp Status"("Waiting for ramp to start..." ("AutoRamp Status")) -> ()
            n258 = local read "ramp start time"() -> (w384:timestamp)
            n259 = Multiply(x=w387, y=60.0) -> (x*y=w385:dbl)
            n260 = Add(x=w385, y=w378) -> (x+y=w383:dbl)
            n261 = Add(x=w383, y=w384) -> (x+y=w382:timestamp)
            n262 = Multiply(x=w372, y=60.0) -> (x*y=w373:dbl)
            n263 = Add(x=w382, y=w375) -> (x+y=w381:timestamp)
            n264 = local write "ramp down start time"(w382) -> ()
            n265 = Add(x=w381, y=w373) -> (x+y=w380:timestamp)
            n266 = local write "ramp finish time"(w380) -> ()
          }
        }
      }
      frame "Calculate ramp time" {
        n267 = local read "Ramp down rate (mA/s)"() -> (w426:dbl)
        n268 = local read "Max current (A)"() -> (w433:dbl)
        n269 = local read "Ramp up rate (mA/s)"() -> (w430:dbl)
        n270 = local read "Timeout (ms)"() -> (w445:i32)
        n271 = local read "Timeout (ms)"() -> (w440:i32)
        n272 = local read "Max current (A)"() -> (w427:dbl)
        n273 = Divide(x=w445, y=1000) -> (x/y=w443:dbl)
        n274 = Multiply(x=w433, y=1000.0) -> (x*y=w431:dbl)
        n275 = Divide(x=w440, y=1000) -> (x/y=w442:dbl)
        n276 = Multiply(x=w427, y=1000.0) -> (x*y=w429:dbl)
        n277 = Divide(x=w431, y=w430) -> (x/y=w416:dbl)
        n278 = Multiply(x=w430, y=w443) -> (x*y=w435:dbl)
        n279 = Multiply(x=w426, y=w442) -> (x*y=w434:dbl)
        n280 = Divide(x=w429, y=w426) -> (x/y=w413:dbl)
        n281 = Divide(x=w434, y=10.0) -> (x/y=w437:dbl)
        n282 = Divide(x=w435, y=10.0) -> (x/y=w436:dbl)
        n283 = local write "Ramp down step size (mA)"(w434) -> ()
        n284 = local write "Ramp up step size (mA)"(w435) -> ()
        n285 = Divide(x=w413, y=60.0) -> (x/y=w414:dbl)
        n286 = local write "Ramp down step size (%)"(w437) -> ()
        n287 = local write "Ramp up step size (%)"(w436) -> ()
        n288 = local write "ramp down time (min)"(w414) -> ()
        n289 = Divide(x=w416, y=60.0) -> (x/y=w417:dbl)
        n290 = local write "ramp up time (min)"(w417) -> ()
        n291 = local read "soak time (minutes)"() -> (w425:dbl)
        n292 = local read "delay after ramp down (min)"() -> (w411:dbl)
        n293 = Multiply(x=w425, y=60.0) -> (x*y=w423:dbl)
        n294 = Add(x=w423, y=w416) -> (x+y=w421:dbl)
        n295 = Add(x=w421, y=w413) -> (x+y=w422:dbl)
        n296 = Multiply(x=60.0, y=w411) -> (x*y=w410:dbl)
        n297 = Add(x=w422, y=w410) -> (x+y=w420:dbl)
        n298 = Divide(x=w420, y=60.0) -> (x/y=w418:dbl)
        n299 = local write "cycle time (min)"(w418) -> ()
      }
      frame "autoramp" {
        n300 = local read "current time"() -> (w448:timestamp)
        n301 = local read "ramp start time"() -> (w447:timestamp)
        n302 = Greater?(x=w448, y=w447) -> (0:w446:bool)
        n303 = case shown="True" w446 {
          frame False {
            n304 = local write "Ramp Status"("waiting for ramp start time" ("AutoRamp Status")) -> ()
          }
          frame True {
            n305 = local read "ramp down start time"() -> (w452:timestamp)
            n306 = local read "current time"() -> (w451:timestamp)
            n307 = Greater?(x=w451, y=w452) -> (0:w450:bool)
            n308 = case shown="False" w450 {
              frame False {
                n309 = local read "Max current (A)"() -> (w454:dbl)
                n310 = local read "Magnet Current (A)"() -> (w455:dbl)
                n311 = Greater Or Equal?(x=w455, y=w454) -> (x >= y?=w453:bool)
                n312 = case shown="False" w453 {
                  frame False {
                    n313 = local read "Ramp Magnet Up"() -> (w458:bool)
                    n314 = Equal?(x=w458, y=TRUE) -> (x = y?=w456:bool)
                    n315 = case shown="False" w456 {
                      frame False {
                        n316 = property on="Ramp Magnet Up" class="Bool (strict)"("Val(Sgnl)"=TRUE ("Value (Signaling)")) -> ()  [unwired: 2 in, 2 out]
                        n317 = property on="Heat Switch" class="Bool (strict)"("Val(Sgnl)"=TRUE ("Value (Signaling)")) -> ()  [unwired: 2 in, 2 out]
                      }
                      frame True {
                      }
                    }
                    n318 = local write "Ramp Status"("ramping up" ("AutoRamp Status")) -> ()
                  }
                  frame True {
                    n319 = local write "Ramp Magnet Up"(FALSE ("Auto-Ramp")) -> ()
                    n320 = local write "Ramp Status"("soaking" ("AutoRamp Status")) -> ()
                  }
                }
              }
              frame True {
                n321 = local read "Max current (A)"() -> (w465:dbl)
                n322 = local read "Magnet Current (A)"() -> (w466:dbl)
                n323 = Greater Or Equal?(x=w466, y=w465) -> (x >= y?=w464:bool)
                n324 = case shown="False" w464 {
                  frame False {
                    n325 = local read "Magnet Current (A)"() -> (w469:dbl)
                    n326 = local read "Ramp down step size (mA)"() -> (w471:dbl)
                    n327 = local write "Ramp Status"("ramping down" ("AutoRamp Status")) -> ()
                    n328 = Multiply(x=w469, y=1000.0) -> (x*y=w467:dbl)
                    n329 = Greater Or Equal?(x=w467, y=w471) -> (x >= y?=w470:bool)
                    n330 = case shown="False" w470 {
                      frame False {
                        n331 = local write "Auto-Ramp"(FALSE ("Auto-Ramp")) -> ()
                      }
                      frame True {
                      }
                    }
                  }
                  frame True {
                    n332 = property on="Ramp Magnet Down" class="Bool (strict)"("Val(Sgnl)"=TRUE ("Value (Signaling)")) -> ()  [unwired: 2 in, 2 out]
                    n333 = property on="Heat Switch" class="Bool (strict)"("Val(Sgnl)"=FALSE ("Value (Signaling)")) -> ()  [unwired: 2 in, 2 out]
                    n334 = local write "Ramp Status"("ramping down" ("Ramp Status")) -> ()
                  }
                }
              }
            }
          }
        }
      }
      frame "check ramp state" {
        n335 = local read "Ramp State"() -> (w478:u16)
        n336 = case shown="2" w478 {
          tunnel: w477 -> [_ _ w527 _ _ _ _]
          frame 0 {
            # "Ramp Up"
            # "Steps:\n1. Increment magnet until max value is reached\n2. Change Ramp State to Soak (hold)"
            n337 = local read "Magnet Current (A)"() -> (w481:dbl)
            n338 = local read "Max current (A)"() -> (w480:dbl)
            n339 = Greater Or Equal?(x=w481, y=w480) -> (x >= y?=w479:bool)
            n340 = case shown="False" w479 {
              frame False {
                w495 = u16 0 items=["sample heater", "output 1 (warm-up heater) ", "output 2 (analog/still)"] ("Output (0: sample heater)")
                # "increment magnet"
                n341 = local read "Ramp up rate (mA/s)"() -> (w493:dbl)
                n342 = local read "Timeout (ms)"() -> (w492:i32)
                n343 = local read "Magnet Current Multiplier"() -> (w482:dbl)
                n344 = local read "Heater Range Actual"() -> (w485:u16)
                n345 = Divide(x=w492, y=1000) -> (x/y=w490:dbl)
                n346 = Multiply(x=w493, y=w490) -> (x*y=w483:dbl)
                n347 = Divide(x=w483, y=w482) -> (x/y=w484:dbl)
                n348 = local write "Ramp up step size (mA)"(w483) -> ()
                n349 = local read "Magnet Current (%)"() -> (w487:dbl)
                n350 = case shown="1" w485 {
                  tunnel: [w497 w500 w503 w506 w509 w512 w515 w518 w521] -> w486
                  tunnel: w484 -> [w496 w499 w502 w505 w508 w511 w514 w517 w520]
                  frame 2 {
                    n351 = Divide(x=w496, y=10.0) -> (x/y=w497:dbl)
                  }
                  frame 3 {
                    n352 = Divide(x=w499, y=31.6) -> (x/y=w500:dbl)
                  }
                  frame 4 {
                    n353 = Divide(x=w502, y=100.0) -> (x/y=w503:dbl)
                  }
                  frame 5 {
                    n354 = Divide(x=w505, y=316.0) -> (x/y=w506:dbl)
                  }
                  frame 6 {
                    n355 = Divide(x=w508, y=1000.0) -> (x/y=w509:dbl)
                  }
                  frame 7 {
                    n356 = Divide(x=w511, y=3160.0) -> (x/y=w512:dbl)
                  }
                  frame 8 {
                    n357 = Divide(x=w514, y=10000.0) -> (x/y=w515:dbl)
                  }
                  frame 0, Default {
                    n358 = Multiply(x=w517, y=0.0) -> (x*y=w518:dbl)
                  }
                  frame 1 {
                    n359 = Divide(x=w520, y=3.16) -> (x/y=w521:dbl)
                  }
                }
                n360 = local read "Heater Range Set"() -> (w489:u16)
                n361 = Add(x=w487, y=w486) -> (x+y=w494:dbl)
                n362 = local read "ls372"() -> (w488:refnum<visa-resource-name>)
                n363 = call "Configure Control Parameters.vi"("VISA resource name"=w488, "Output (0: sample heater)"=w495, "Manual Output (0.000%)"=w494, "Heater Range (0: Off)"=w489) -> ()  [unwired: 10 in, 2 out]
              }
              frame True {
                w524 = u16 1 items=["Ramp Up", "Soak (hold)", "Ramp Down", "Ramp up to Setpoint", "Closed Loop Feedback", "Ramp down from Setpoint", "Magnet off"] ("Ramp State")
                n364 = local write "Ramp State"(w524) -> ()
                n365 = local write "Ramp Magnet Up"(FALSE ("Ramp Magnet Up")) -> ()
              }
            }
          }
          frame 1, Default {
            # "Soak (hold)"
            # "Steps:\n1. Do nothing! but indicate that magnet is on"
            n366 = local write "Magnet Current Multiplier"(25.66 ("Magnet Current Multiplier")) -> ()
          }
          frame 2 {
            # "Steps:\n1. Decrement magnet until min value is reached\n2. Change Ramp State to Magnet off"
            # "Ramp Down"
            n367 = local read "Ramp up step size (mA)"() -> (w529:dbl)
            n368 = local read "Magnet Current (A)"() -> (w531:dbl)
            n369 = Divide(x=w529, y=1000.0) -> (x/y=w530:dbl)
            n370 = Less Or Equal?(x=w531, y=w530) -> (x <= y?=w526:bool)
            n371 = case shown="True" w526 {
              tunnel: w527 -> [_ w582]
              frame False {
                w545 = u16 0 items=["sample heater", "output 1 (warm-up heater) ", "output 2 (analog/still)"] ("Output (0: sample heater)")
                n372 = local read "Ramp down rate (mA/s)"() -> (w542:dbl)
                n373 = local read "Magnet Current Multiplier"() -> (w532:dbl)
                n374 = local read "Timeout (ms)"() -> (w541:i32)
                n375 = local read "Heater Range Actual"() -> (w535:u16)
                n376 = Divide(x=w541, y=1000) -> (x/y=w539:dbl)
                n377 = Multiply(x=w542, y=w539) -> (x*y=w533:dbl)
                n378 = local read "Magnet Current (%)"() -> (w537:dbl)
                n379 = local write "Ramp down step size (mA)"(w533) -> ()
                n380 = Divide(x=w533, y=w532) -> (x/y=w534:dbl)
                n381 = case shown="2" w535 {
                  tunnel: [w547 w550 w553 w556 w559 w562 w565 w568 w571] -> w536
                  tunnel: w534 -> [w546 w549 w552 w555 w558 w561 w564 w567 w570]
                  frame 2 {
                    n382 = Divide(x=w546, y=10.0) -> (x/y=w547:dbl)
                  }
                  frame 3 {
                    n383 = Divide(x=w549, y=31.6) -> (x/y=w550:dbl)
                  }
                  frame 4 {
                    n384 = Divide(x=w552, y=100.0) -> (x/y=w553:dbl)
                  }
                  frame 5 {
                    n385 = Divide(x=w555, y=316.0) -> (x/y=w556:dbl)
                  }
                  frame 6 {
                    n386 = Divide(x=w558, y=1000.0) -> (x/y=w559:dbl)
                  }
                  frame 7 {
                    n387 = Divide(x=w561, y=3160.0) -> (x/y=w562:dbl)
                  }
                  frame 8 {
                    n388 = Divide(x=w564, y=10000.0) -> (x/y=w565:dbl)
                  }
                  frame 0, Default {
                    n389 = Multiply(x=w567, y=0.0) -> (x*y=w568:dbl)
                  }
                  frame 1 {
                    n390 = Divide(x=w570, y=3.16) -> (x/y=w571:dbl)
                  }
                }
                n391 = Subtract(x=w537, y=w536) -> (x-y=w543:dbl)
                n392 = local read "Heater Range Set"() -> (w538:u16)
                n393 = local read "ls372"() -> (w544:refnum<visa-resource-name>)
                n394 = call "Configure Control Parameters.vi"("VISA resource name"=w544, "Output (0: sample heater)"=w545, "Manual Output (0.000%)"=w543, "Heater Range (0: Off)"=w538) -> ()  [unwired: 10 in, 2 out]
              }
              frame True {
                n395 = local read "delay after ramp down (min)"() -> (w575:dbl)
                n396 = local read "Timeout (ms)"() -> (w580:i32)
                n397 = Divide(x=w580, y=1000) -> (x/y=w578:dbl)
                n398 = Multiply(x=w575, y=60.0) -> (x*y=w574:dbl)
                n399 = Divide(x=w574, y=w578) -> (x/y=w581:dbl)
                n400 = local read "counter"() -> (w576:dbl)
                n401 = Greater Or Equal?(x=w576, y=w581) -> (x >= y?=w577:bool)
                n402 = case shown="True" w577 {
                  tunnel: w582 -> [_ w595]
                  tunnel: w576 -> [w583 _]
                  frame False {
                    n403 = Increment(x=w583) -> (x+1=w584:dbl)
                    n404 = local write "counter"(w584) -> ()
                  }
                  frame True {
                    w585 = u16 0 items=["Off", "31.6 uA", "100 uA", "316 uA", "1.00 mA", "3.16 mA", "10.0 mA", "31.6 mA", "100 mA"] ("Heater Range Set")
                    w589 = u16 0 items=["Off", "On", "Alarms", "Sample Heater Zone", "Warmup Heater Zone"] ("Relay Mode (0: Off)")
                    w594 = u16 0 items=["unipolar", "bipolar"] ("polarity")
                    w600 = u16 0 items=["sample heater", "output 1 (warm-up heater) ", "output 2 (analog/still)"] ("Output (0: sample heater)")
                    w598 = u16 0 items=["off", "monitor out", "open loop (manual)", "zone", "still", "closed loop (PID)", "warmup"] ("mode")
                    n405 = local write "Ramp Status"("Ramp finished. " ("AutoRamp Status")) -> ()
                    n406 = local read "control channel"() -> (w590:string)
                    n407 = local read "End of Ramp Temp Control"() -> (w596:bool)
                    n408 = local write "Magnet Current Multiplier"(0.1 ("Magnet Current Multiplier")) -> ()
                    n409 = local write "Ramp Magnet Down"(FALSE ("Auto-Ramp")) -> ()
                    n410 = local read "ls372"() -> (w599:refnum<visa-resource-name>)
                    n411 = call "configure heater output.vi"("VISA resource name"=w599, "power up enable"=FALSE, "polarity"=w594, "delay"=0, "Output (0: sample heater)"=w600, "mode"=w598, "input/channel"=w590, "filter"=FALSE) -> ("VISA resource name out"=w588:refnum<visa-resource-name>, "error out"=w587:errorcluster)  [unwired: 6 in]
                    n412 = call "Configure Relays.vi"("Relay Mode (0: Off)"=w589, "error in (no error)"=w587, "VISA resource name"=w588) -> ()  [unwired: 7 in, 2 out]
                    n413 = case shown="False" w596 {
                      tunnel: w595 -> [_ w605]
                      frame False {
                        w603 = u16 6 items=["Ramp Up", "Soak (hold)", "Ramp Down", "Ramp up to Setpoint", "Closed Loop Feedback", "Ramp down from Setpoint", "Magnet off"] ("Ramp State")
                        n414 = local write "Ramp State"(w603) -> ()
                        n415 = local write "Manual temp control"(FALSE ("temp control?")) -> ()
                      }
                      frame True {
                        n416 = Enqueue Element(queue=w605, element="turn on PID feedback") -> ()  [unwired: 2 in, 3 out]
                        n417 = local write "Ramp Status"("Turning on PID FEEDBACK\n" ("Arduino Response 2")) -> ()
                      }
                    }
                    n418 = local write "Heater Range Set"(w585) -> ()
                  }
                }
              }
            }
          }
          frame 3 {
            # "Ramp up to Setpoint"
          }
          frame 4 {
            # "Steps:\n1. Keep an eye on magnet value. If magnet runs out, turn it off"
            # "Closed Loop Feedback"
            n419 = local read "Magnet Current (A)"() -> (w609:dbl)
            n420 = Less Or Equal?(x=w609, y=0.003) -> (x <= y?=w607:bool)
            n421 = case shown="False" w607 {
              frame False {
                n422 = local write "counter 2"(0.0 ("counter 2")) -> ()
                n423 = local write "Ramp Status"("controlling..." ("Ramp Status")) -> ()
              }
              frame True {
                n424 = local read "counter 2"() -> (w613:dbl)
                n425 = Greater Or Equal?(x=w613, y=300.0) -> (x >= y?=w612:bool)
                n426 = case shown="False" w612 {
                  tunnel: w613 -> [w615 _]
                  frame False {
                    n427 = Increment(x=w615) -> (x+1=w616:dbl)
                    n428 = local write "counter 2"(w616) -> ()
                  }
                  frame True {
                    w617 = u16 6 items=["Ramp Up", "Soak (hold)", "Ramp Down", "Ramp up to Setpoint", "Closed Loop Feedback", "Ramp down from Setpoint", "Magnet off"] ("Ramp State")
                    w634 = u16 0 items=["Off", "31.6 uA", "100 uA", "316 uA", "1.00 mA", "3.16 mA", "10.0 mA", "31.6 mA", "100 mA"] ("Heater Range (0: Off)")
                    w623 = u16 0 items=["unipolar", "bipolar"] ("polarity")
                    w621 = u16 0 items=["off", "monitor out", "open loop (manual)", "zone", "still", "closed loop (PID)", "warmup"] ("mode")
                    w628 = u16 0 items=["sample heater", "output 1 (warm-up heater) ", "output 2 (analog/still)"] ("Output (0: sample heater)")
                    n429 = local read "ls372"() -> (w630:refnum<visa-resource-name>)
                    n430 = Get Date/Time String() -> (time string=w619:string)  [unwired: 3 in, 1 out]
                    n431 = local write "Ramp State"(w617) -> ()
                    n432 = call "Configure Setpoint.vi"("Setpoint (0.00000E+0)"=0.01, "VISA resource name"=w630) -> ("VISA resource name out"=w631:refnum<visa-resource-name>)  [unwired: 8 in, 1 out]
                    n433 = Concatenate Strings("magnet ran out at " ("Ramp Status"), w619) -> (w620:string)
                    n434 = local read "control channel"() -> (w633:string)
                    n435 = local write "Ramp Status"(w620) -> ()
                    n436 = local write "Heater Range Set"(w634) -> ()
                    n437 = call "configure heater output.vi"("VISA resource name"=w631, "power up enable"=FALSE, "polarity"=w623, "delay"=0, "Output (0: sample heater)"=w628, "mode"=w621, "input/channel"=w633, "filter"=FALSE) -> ("VISA resource name out"=w626:refnum<visa-resource-name>, "error out"=w627:errorcluster)  [unwired: 6 in]
                    n438 = call "Configure Control Parameters.vi"("VISA resource name"=w626, "Output (0: sample heater)"=w628, "Manual Output (0.000%)"=0.0, "Heater Range (0: Off)"=w634, "error in (no error)"=w627) -> ()  [unwired: 9 in, 2 out]
                  }
                }
              }
            }
          }
          frame 5 {
            # "Ramp down from Setpoint"
            n439 = local read "Ramp down step size (mA)"() -> (w637:dbl)
            n440 = local read "Magnet Current (A)"() -> (w639:dbl)
            n441 = Divide(x=w637, y=1000.0) -> (x/y=w638:dbl)
            n442 = Less Or Equal?(x=w639, y=w638) -> (x <= y?=w635:bool)
            n443 = case shown="False" w635 {
              frame False {
                n444 = local read "ls372"() -> (w640:refnum<visa-resource-name>)
                n445 = call "Get Setpoint.vi"("VISA resource name"=w640) -> ("Setpoint (0.00000E+0)"=w643:dbl)  [unwired: 8 in, 2 out]
                n446 = Greater Or Equal?(x=w643, y=0.01) -> (x >= y?=w641:bool)
                n447 = case shown="True" w641 {
                  frame False {
                  }
                  frame True {
                    w659 = u16 0 items=["sample heater", "output 1 (warm-up heater) ", "output 2 (analog/still)"] ("Output (0: sample heater)")
                    w651 = u16 0 items=["unipolar", "bipolar"] ("polarity")
                    w649 = u16 5 items=["off", "monitor out", "open loop (manual)", "zone", "still", "closed loop (PID)", "warmup"] ("mode")
                    w648 = u16 0 items=["sample heater", "output 1 (warm-up heater) ", "output 2 (analog/still)"] ("Output (0: sample heater)")
                    n448 = local read "control channel"() -> (w646:string)
                    n449 = local read "ls372"() -> (w656:refnum<visa-resource-name>)
                    n450 = local read "Heater Range Set"() -> (w647:u16)
                    n451 = call "configure heater output.vi"("VISA resource name"=w656, "power up enable"=FALSE, "polarity"=w651, "delay"=0, "Output (0: sample heater)"=w648, "mode"=w649, "input/channel"=w646, "filter"=FALSE) -> ("VISA resource name out"=w654:refnum<visa-resource-name>, "error out"=w655:errorcluster)  [unwired: 6 in]
                    n452 = call "Configure Control Parameters.vi"("VISA resource name"=w654, "Output (0: sample heater)"=w659, "Manual Output (0.000%)"=0.0, "Heater Range (0: Off)"=w647, "error in (no error)"=w655) -> ("VISA resource name out"=w657:refnum<visa-resource-name>, "error out"=w658:errorcluster)  [unwired: 9 in]
                    n453 = call "Configure Setpoint.vi"("error in (no error)"=w658, "Setpoint (0.00000E+0)"=0.001, "Output (0: Sample Heater)"=w659, "VISA resource name"=w657) -> ()  [unwired: 6 in, 2 out]
                  }
                }
              }
              frame True {
                w664 = u16 0 items=["unipolar", "bipolar"] ("polarity")
                w665 = u16 0 items=["Off", "31.6 uA", "100 uA", "316 uA", "1.00 mA", "3.16 mA", "10.0 mA", "31.6 mA", "100 mA"] ("Heater Range Set")
                w666 = u16 6 items=["Ramp Up", "Soak (hold)", "Ramp Down", "Ramp up to Setpoint", "Closed Loop Feedback", "Ramp down from Setpoint", "Magnet off"] ("Ramp State")
                w670 = u16 0 items=["sample heater", "output 1 (warm-up heater) ", "output 2 (analog/still)"] ("Output (0: sample heater)")
                w668 = u16 0 items=["off", "monitor out", "open loop (manual)", "zone", "still", "closed loop (PID)", "warmup"] ("mode")
                n454 = local write "Ramp Status"("Ramp finished. " ("AutoRamp Status")) -> ()
                n455 = local read "control channel"() -> (w660:string)
                n456 = local read "ls372"() -> (w669:refnum<visa-resource-name>)
                n457 = call "configure heater output.vi"("VISA resource name"=w669, "power up enable"=FALSE, "polarity"=w664, "delay"=0, "Output (0: sample heater)"=w670, "mode"=w668, "input/channel"=w660, "filter"=FALSE) -> ()  [unwired: 6 in, 2 out]
                n458 = local write "Ramp Magnet Down"(FALSE ("Auto-Ramp")) -> ()
                n459 = local write "Heater Range Set"(w665) -> ()
                n460 = local write "Ramp State"(w666) -> ()
              }
            }
          }
          frame 6 {
            # "Magnet off"
            n461 = local read "Heater Range Actual"() -> (w674:u16)
            n462 = Equal?(x=w674, y=u16 0) -> (x = y?=w672:bool)
            n463 = case shown="False" w672 {
              frame False {
                w675 = u16 0 items=["Off", "31.6 uA", "100 uA", "316 uA", "1.00 mA", "3.16 mA", "10.0 mA", "31.6 mA", "100 mA"] ("Heater Range Set")
                n464 = local write "Heater Range Set"(w675) -> ()
              }
              frame True {
              }
            }
          }
        }
      }
      frame "turn on PID feedback" {
        w677 = u16 4 items=["Ramp Up", "Soak (hold)", "Ramp Down", "Ramp up to Setpoint", "Closed Loop Feedback", "Ramp down from Setpoint", "Magnet off"] ("Ramp State")
        w678 = u16 3 items=["Off", "31.6 uA", "100 uA", "316 uA", "1.00 mA", "3.16 mA", "10.0 mA", "31.6 mA", "100 mA"] ("Heater Range (0: Off)")
        w693 = u16 0 items=["sample heater", "output 1 (warm-up heater) ", "output 2 (analog/still)"] ("Output (0: sample heater)")
        w684 = u16 0 items=["unipolar", "bipolar"] ("polarity")
        w682 = u16 5 items=["off", "monitor out", "open loop (manual)", "zone", "still", "closed loop (PID)", "warmup"] ("mode")
        w681 = u16 0 items=["sample heater", "output 1 (warm-up heater) ", "output 2 (analog/still)"] ("Output (0: sample heater)")
        n465 = local read "ls372"() -> (w689:refnum<visa-resource-name>)
        n466 = local read "control channel"() -> (w680:string)
        n467 = local write "counter 2"(0.0 ("counter 2")) -> ()
        n468 = call "configure heater output.vi"("VISA resource name"=w689, "power up enable"=FALSE, "polarity"=w684, "delay"=0, "Output (0: sample heater)"=w681, "mode"=w682, "input/channel"=w680, "filter"=FALSE) -> ("VISA resource name out"=w687:refnum<visa-resource-name>, "error out"=w688:errorcluster)  [unwired: 6 in]
        n469 = call "Configure Control Parameters.vi"("VISA resource name"=w687, "Output (0: sample heater)"=w693, "Manual Output (0.000%)"=0.0, "Heater Range (0: Off)"=w678, "error in (no error)"=w688) -> ("VISA resource name out"=w690:refnum<visa-resource-name>, "error out"=w691:errorcluster)  [unwired: 9 in]
        n470 = local read "setpoint (K)"() -> (w692:dbl)
        n471 = local write "Ramp State"(w677) -> ()
        n472 = local write "Heater Range Set"(w678) -> ()
        n473 = call "Configure Setpoint.vi"("error in (no error)"=w691, "Setpoint (0.00000E+0)"=w692, "Output (0: Sample Heater)"=w693, "VISA resource name"=w690) -> ()  [unwired: 6 in, 2 out]
      }
      frame "Write LS372 Settings" {
        w694 = u16 1 items=["Kelvin"=1, "Ohms"=2] ("Preferred Units (2: Ohms)")
        n474 = local read "ls372"() -> (w702:refnum<visa-resource-name>)
        n475 = call "Configure Input Sensor Range.vi"("VISA resource name"=w702, "Channel (1)"="Channel (1)", "Excitation Mode (0: Voltage)"="Excitation Mode (0: Voltage)", "Excitation Range (5: 200 uV / 100 pA)"="Excitation Range (5: 200 uV / 100 pA)", "Autorange (0: Autorange off)"="Autorange (0: Autorange off)", "Resistance Range (17: 200 kOhm)"="Resistance Range (17: 200 kOhm)", "Excitation  (T: On)"="Excitation  (T: On)", "Preferred Units (2: Ohms)"=w694, "Temperature Limit (0 Kelvin)"=0.0) -> ()  [unwired: 9 in, 2 out]
      }
      frame "Warmup Heater" {
        n476 = local read "ls372"() -> (w705:refnum<visa-resource-name>)
        n477 = call "LS372_warmup_heater.vi"("Heater ON/OFF"="Heater ON/OFF", "Warmup Heater Power (W)"="Warmup Heater Power (W)", "VISA resource name"=w705) -> ()  [unwired: 7 in, 2 out]
      }
    }
    n478 = Get Queue Status(queue=w46) -> (# elements in queue=w51:i32)  [unwired: 2 in, 7 out]
    n479 = Equal?(x=w51, y=0) -> (x = y?=w48:bool)
    n480 = local read "stopping"() -> (w49:bool)
    n481 = And(x=w49, y=w48) -> (x .and. y?=w47:bool)
  }
  n482 = while {
    tunnel: w43 -> [w709]
    tunnel: [w707] -> _
    stop <- w708 stop-if-true
    n483 = local read "Timeout (ms)"() -> (w706:i32)
    n484 = event shown="[2] \"initialize\": Value Change" {
      selector: _ -> [_ _ _ _ _ _ _ _ _ _ _ _]
      dyn-events: _ -> [_ _ _ _ _ _ _ _ _ _ _ _]
      timeout: w706 -> [_ _ _ _ _ _ _ _ _ _ _ _]
      tunnel: w709 -> [w731 w748 w753 w775 w781 w790 w801 w802 w827 w829 w831 w840]
      tunnel: [_ _ _ _ _ _ _ _ _ _ _ w832] -> w707
      event Timeout {
        # "normal operating mode"
        # "record temps after\nevery # seconds"
        n485 = event-data() -> ()  [unwired: 1 in, 3 out]
        n486 = local read "Read LS336"() -> (w728:bool)
        n487 = local read "Read LS372"() -> (w727:bool)
        n488 = Get Date/Time In Seconds() -> (seconds since 1Jan1904=w723:timestamp)
        n489 = case shown="True" w728 {
          tunnel: w731 -> [w738 w742]
          tunnel: [w738 w740] -> w730
          frame False {
          }
          frame True {
            n490 = Enqueue Element(queue=w742, element="336 read temp") -> (queue out=w741:refnum<queue>)  [unwired: 2 in, 2 out]
            n491 = Enqueue Element(queue=w741, element="336 read R") -> (queue out=w740:refnum<queue>)  [unwired: 2 in, 2 out]
          }
        }
        n492 = case shown="True" w727 {
          tunnel: w730 -> [w744 w747]
          tunnel: [w744 w745] -> w729
          frame False {
          }
          frame True {
            n493 = Enqueue Element(queue=w747, element="372 read temp") -> (queue out=w745:refnum<queue>)  [unwired: 2 in, 2 out]
          }
        }
        n494 = To Double Precision Float(number=w723) -> (double precision float=w724:dbl)
        n495 = Quotient & Remainder(x=w724, y=10.0) -> (x-y*floor(x/y)=w721:dbl)  [unwired: 1 out]
        n496 = Round Toward -Infinity(1:w721) -> (0:w718:dbl)
        n497 = Equal?(x=w718, y=0.0) -> (x = y?=w719:bool)
        n498 = And(x="Record Temps", y=w719) -> (x .and. y?=w717:bool)
        n499 = case shown="False" w717 {
          tunnel: w729 -> [w734 w737]
          tunnel: [w734 w736] -> w726
          tunnel: "record temps" ("element") -> [_ w735]
          frame False {
          }
          frame True {
            n500 = Enqueue Element(queue=w737, element=w735) -> (queue out=w736:refnum<queue>)  [unwired: 2 in, 2 out]
          }
        }
        n501 = Get Date/Time In Seconds() -> (seconds since 1Jan1904=→"current time":timestamp)
        n502 = local read "Auto-Ramp"() -> (w711:bool)
        n503 = Enqueue Element(queue=w726, element="read current") -> (queue out=w713:refnum<queue>)  [unwired: 2 in, 2 out]
        n504 = Enqueue Element(queue=w713, element="check ramp state") -> (queue out=w710:refnum<queue>)  [unwired: 2 in, 2 out]
        n505 = case shown="False" w711 {
          tunnel: w710 -> [_ w732]
          frame False {
          }
          frame True {
            n506 = Enqueue Element(queue=w732, element="autoramp") -> ()  [unwired: 2 in, 3 out]
          }
        }
      }
      event "Auto-Ramp": Value Change {
        n507 = event-data() -> ("NewVal"=w749:bool)  [unwired: 1 in, 5 out]
        n508 = case shown="True" w749 {
          tunnel: w748 -> [_ w751]
          frame False {
          }
          frame True {
            n509 = Enqueue Element(queue=w751, element="set up autoramp times") -> ()  [unwired: 2 in, 3 out]
          }
        }
      }
      event "initialize": Value Change {
        # "program starts here. this sets up connections to lakeshore monitors"
        n510 = event-data() -> ()  [unwired: 1 in, 3 out]
        n511 = local read "Read LS336"() -> (w759:bool)
        n512 = local write "Ramp Magnet Up"(FALSE ("Ramp Magnet Up")) -> ()
        n513 = local write "Ramp Magnet Down"(FALSE ("Ramp Magnet Down")) -> ()
        n514 = local write "Auto-Ramp"(FALSE ("Ramp Magnet Down")) -> ()
        n515 = case shown="True" w759 {
          tunnel: [errorcluster {"status"=FALSE, "code"=0, "source"=""} ("error out") w771] -> w758
          frame False {
          }
          frame True {
            # "open/close the visa\nconnection to aviod\nerrors after rebooting\nthe 336. Dunno why\nit works. CB"
            n516 = local read "ls336"() -> (w767:refnum<visa-resource-name>)
            n517 = VISA Open(VISA resource name=w767) -> (VISA resource name=w769:refnum<visa-resource-name>, error out=w770:errorcluster)  [unwired: 4 in]
            n518 = VISA Close(VISA resource name=w769, error in (no error)=w770) -> (error out=w768:errorcluster)
            n519 = call "Initialize.vi"("error in (no error)"=w768, "Reset (True)"=FALSE, "ID Query (True)"=TRUE, "VISA resource name"=w767) -> ("error out"=w771:errorcluster)  [unwired: 6 in, 1 out]
          }
        }
        n520 = local read "Read LS372"() -> (w755:bool)
        n521 = Enqueue Element(queue=w753, element="check arduino ID") -> ()  [unwired: 2 in, 3 out]
        n522 = case shown="True" w755 {
          tunnel: w758 -> [w760 w763]
          tunnel: [w760 w761] -> _
          frame False {
          }
          frame True {
            n523 = local read "ls372"() -> (w762:refnum<visa-resource-name>)
            n524 = call "Initialize.vi"("error in (no error)"=w763, "Reset (True)"=FALSE, "ID Query (True)"=TRUE, "VISA resource name"=w762) -> ("error out"=w761:errorcluster)  [unwired: 6 in, 1 out]
          }
        }
      }
      event "Heat Switch": Value Change {
        # "Open or close the heat switch"
        n525 = event-data() -> ("NewVal"=w774:bool)  [unwired: 1 in, 5 out]
        n526 = case shown="True" w774 {
          tunnel: w775 -> [w777 w779]
          frame False {
            # "open heat switch"
            n527 = Enqueue Element(queue=w777, element="open heat switch") -> ()  [unwired: 2 in, 3 out]
          }
          frame True {
            # "close heat switch"
            n528 = Enqueue Element(queue=w779, element="close heat switch") -> ()  [unwired: 2 in, 3 out]
          }
        }
      }
      event "Ramp Magnet Up": Value Change {
        n529 = event-data() -> ("NewVal"=w780:bool)  [unwired: 1 in, 5 out]
        n530 = case shown="True" w780 {
          tunnel: w781 -> [_ w788]
          frame False {
            w783 = u16 1 items=["Ramp Up", "Soak (hold)", "Ramp Down", "Ramp up to Setpoint", "Closed Loop Feedback", "Ramp down from Setpoint", "Magnet off"] ("Ramp State")
            n531 = local write "Ramp Status"("holding" ("Ramp Status")) -> ()
            n532 = local write "Ramp State"(w783) -> ()
          }
          frame True {
            w785 = u16 2 items=["Off", "31.6 uA", "100 uA", "316 uA", "1.00 mA", "3.16 mA", "10.0 mA", "31.6 mA", "100 mA"] ("Heater Range (0: Off)")
            w786 = u16 0 items=["Ramp Up", "Ramp Down", "Ramp up to Setpoint", "Ramp down from Setpoint", "Closed Loop Feedback", "Soak (hold)"] ("Ramp State")
            n533 = local write "Ramp State"(w786) -> ()
            n534 = local write "Ramp Status"("ramping up" ("Ramp Status")) -> ()
            n535 = local write "Heater Range Set"(w785) -> ()
            n536 = Enqueue Element(queue=w788, element="initialize ramp up") -> ()  [unwired: 2 in, 3 out]
          }
        }
      }
      event "Ramp Magnet Down": Value Change {
        n537 = event-data() -> ("NewVal"=w789:bool)  [unwired: 1 in, 5 out]
        n538 = case shown="True" w789 {
          tunnel: w790 -> [_ _]
          frame True {
            n539 = local read "Ramp State"() -> (w792:u16)
            n540 = case shown="0, Default" w792 {
              frame 0, Default {
                w795 = u16 2 items=["Ramp Up", "Soak (hold)", "Ramp Down", "Ramp up to Setpoint", "Closed Loop Feedback", "Ramp down from Setpoint", "Magnet off"] ("Ramp State")
                n541 = local write "Ramp State"(w795) -> ()
                n542 = local write "Ramp Magnet Up"(FALSE ("Ramp Magnet Up")) -> ()
              }
              frame 4 {
                w796 = u16 5 items=["Ramp Up", "Soak (hold)", "Ramp Down", "Ramp up to Setpoint", "Closed Loop Feedback", "Ramp down from Setpoint", "Magnet off"] ("Ramp State")
                n543 = local write "Ramp State"(w796) -> ()
              }
              frame 5 {
                w797 = u16 5 items=["Ramp Up", "Soak (hold)", "Ramp Down", "Ramp up to Setpoint", "Closed Loop Feedback", "Ramp down from Setpoint", "Magnet off"] ("Ramp State")
                n544 = local write "Ramp State"(w797) -> ()
              }
              frame 6 {
              }
            }
            n545 = local write "Ramp Status"("ramping down" ("Ramp Status")) -> ()
            n546 = local write "counter"(0.0 ("counter")) -> ()
          }
          frame False {
            w798 = u16 1 items=["Ramp Up", "Soak (hold)", "Ramp Down", "Ramp up to Setpoint", "Closed Loop Feedback", "Ramp down from Setpoint", "Magnet off"] ("Ramp State")
            n547 = local write "Ramp State"(w798) -> ()
            n548 = local write "Ramp Status"("holding" ("Ramp Status")) -> ()
          }
        }
      }
      event "Heater ON/OFF", "Warmup Heater Power (W)": Value Change {
        n549 = event-data() -> ()  [unwired: 1 in, 6 out]
        n550 = Enqueue Element(queue=w801, element="Warmup Heater") -> ()  [unwired: 2 in, 3 out]
      }
      event "Manual temp control": Value Change {
        n551 = event-data() -> ("NewVal"=w803:bool)  [unwired: 1 in, 5 out]
        n552 = case shown="True" w803 {
          tunnel: w802 -> [_ w819]
          frame False {
            w804 = u16 0 items=["Off", "31.6 uA", "100 uA", "316 uA", "1.00 mA", "3.16 mA", "10.0 mA", "31.6 mA", "100 mA"] ("Heater Range (0: Off)")
            w815 = u16 0 items=["unipolar", "bipolar"] ("polarity")
            w817 = u16 0 items=["off", "monitor out", "open loop (manual)", "zone", "still", "closed loop (PID)", "warmup"] ("mode")
            w810 = u16 0 items=["sample heater", "output 1 (warm-up heater) ", "output 2 (analog/still)"] ("Output (0: sample heater)")
            n553 = local read "ls372"() -> (w808:refnum<visa-resource-name>)
            n554 = call "Configure Setpoint.vi"("Setpoint (0.00000E+0)"=0.01, "VISA resource name"=w808) -> ("VISA resource name out"=w807:refnum<visa-resource-name>)  [unwired: 8 in, 1 out]
            n555 = local read "control channel"() -> (w805:string)
            n556 = local write "Heater Range Set"(w804) -> ()
            n557 = call "configure heater output.vi"("VISA resource name"=w807, "power up enable"=FALSE, "polarity"=w815, "delay"=0, "Output (0: sample heater)"=w810, "mode"=w817, "input/channel"=w805, "filter"=FALSE) -> ("VISA resource name out"=w812:refnum<visa-resource-name>, "error out"=w811:errorcluster)  [unwired: 6 in]
            n558 = call "Configure Control Parameters.vi"("VISA resource name"=w812, "Output (0: sample heater)"=w810, "Manual Output (0.000%)"=0.0, "Heater Range (0: Off)"=w804, "error in (no error)"=w811) -> ()  [unwired: 9 in, 2 out]
          }
          frame True {
            # "if temp is > 500 mK, do nothing"
            n559 = local read "FAA RO600"() -> (w821:dbl)
            n560 = Less?(x=w821, y=0.5) -> (x < y?=w818:bool)
            n561 = case shown="True" w818 {
              tunnel: w819 -> [_ w824]
              frame False {
                n562 = local write "Manual temp control"(FALSE ("temp control?")) -> ()
              }
              frame True {
                n563 = Enqueue Element(queue=w824, element="turn on PID feedback") -> ()  [unwired: 2 in, 3 out]
              }
            }
          }
        }
      }
      event "Check Arduino": Value Change {
        n564 = event-data() -> ()  [unwired: 1 in, 6 out]
        n565 = Enqueue Element(queue=w827, element="check arduino ID") -> ()  [unwired: 2 in, 3 out]
        n566 = local write "Arduino Response"("checking" ("Arduino Response")) -> ()
      }
      event "Calculate Autoramp Time": Value Change {
        n567 = event-data() -> ()  [unwired: 1 in, 6 out]
        n568 = Enqueue Element(queue=w829, element="Calculate ramp time") -> ()  [unwired: 2 in, 3 out]
      }
      event "Excitation Range (5: 200 uV / 100 pA)", "Autorange (0: Autorange off)", "Excitation  (T: On)": Value Change {
        n569 = event-data() -> ()  [unwired: 1 in, 6 out]
        n570 = Enqueue Element(queue=w831, element="Write LS372 Settings") -> ()  [unwired: 2 in, 3 out]
      }
      event "Stop": Value Change {
        # "program ends here. flush queue, close connections to lakeshores"
        n571 = event-data() -> ()  [unwired: 1 in, 3 out]
        n572 = Flush Queue(queue=w840) -> (queue out=w835:refnum<queue>, error out=w834:errorcluster)  [unwired: 1 in, 1 out]
        n573 = Enqueue Element At Opposite End(queue=w835, element="False", error in (no error)=w834) -> (queue out=w837:refnum<queue>, error out=w833:errorcluster)  [unwired: 1 in, 1 out]
        n574 = Enqueue Element At Opposite End(queue=w837, element="False", error in (no error)=w833) -> (queue out=w832:refnum<queue>)  [unwired: 1 in, 2 out]
        n575 = local write "stopping"(TRUE ("cancelling")) -> ()
      }
    }
    n576 = local read "stopping"() -> (w708:bool)
  }
  "stopping" <- FALSE
  "GGG RO600" <- 0.0 ("1K RO600")
  "Magnet RTD" <- 0.0 ("Magnet RTD")
  "4K Diode" <- 0.0 ("4K Diode")
  "77K Diode" <- 0.0 ("77K Diode")
  "FAA RO600" <- 0.0 ("ADR RO600")
  "Sample RuOx" <- 0.0 ("Sample RuOx")
  "GGG RO600 R" <- 0.0 ("1K RO600")
  "Magnet RTD R" <- 0.0 ("Magnet RTD")
  "FAA RO600 R" <- 0.0 ("ADR RO600")
  "Sample RuOx R" <- 0.0 ("Sample RuOx")
  "Magnetic Field (kG)" <- 0.0 ("Magnet Field")
  "Ramp Status" <- "No Action" ("AutoRamp Status")
  "ramp up time (min)" <- 0.0 ("ramp up time (s)")
  "ramp down time (min)" <- 0.0 ("ramp down time (s)")
  "Arduino Response" <- "" ("Arduino Response")
  "Arduino OK" <- FALSE ("Arduino OK")
  "Magnet Current Multiplier" <- 0.1 ("Magnet Current Multiplier")
  "counter" <- 0.0 ("x")
  "counter 2" <- 0.0 ("counter 2")
  "Reading 336" <- FALSE ("Reading 336")
  "Reading 372" <- FALSE ("Reading 372")
  "Heater Range OK" <- FALSE ("Heater Range OK")
